vi "amoure_fast_panel.vi"() -> ()   [LabVIEW 2016]
uses:
  <vilib>/Utility/error.llb/DialogType.ctl
  states/InitializationStates.ctl
  states/DataAcqStates.ctl
  <vilib>/registry/registry.llb/Registry RtKey.ctl
  <vilib>/registry/registry.llb/Registry SAM.ctl
  <vilib>/Utility/error.llb/whitespace.ctl
  <vilib>/Analysis/baseanly.llb/Mean (DBL).vi
  <vilib>/registry/registry.llb/Read Registry Value Simple STR.vi
  Instance           5 11Saved   VFP .vi
  Instance          20 11Saved   VFP .vi
  Instance           6 11Saved   VFP .vi
  Instance          21 11Saved   VFP .vi
  Instance           8 11Saved   VFP .vi
  <vilib>/Analysis/NI_AALPro.lvlib
  <vilib>/Analysis/NI_AALBase.lvlib
panel:
  out "Target Golovochenko  (MOhm)":dbl
  in  "Applied Voltage (V)":dbl
  out "Pore Resistance":dbl
  out "Target Resistance \n(MOhm)":dbl
  out "Membrane-Solution Resistivity":dbl
  out "Membrane Resistance (MOhm)":dbl
  out "Capillary Resistance":dbl
  out "Capillary Diameter":dbl
  in  "Bare Resistance \n(MOhm)":dbl
  out "XY Graph":cluster{"type":sgl[], "type":sgl[]}(graph)
  out "Recording IV":bool
  in  "Start/Stop Saving":bool
  in  "Pick a new filename":bool
  out "Control Amp Overload":bool caption="CA"
  out "Current Overload":bool caption="I"
  out "Voltage Overload":bool caption="V"
  in  "Legacy Save":bool
  out "Front Panel Window:Title 2":string="Gamry Instruments Virtual Front Panel"
  out "Log File Refnum 2":refnum<file>
  in  "Log File 2":path
  in  "Enable Section":bool
  in  "Desired Pore Size (nm)":dbl
  in  "Membrane Thickness \n(nm)":dbl
  in  "Sealed Resistance\n(MOhm)":dbl
  in  "Solution Conductance":dbl
  in  "Smoothing Parameter":i32=100
  out "Resistance (MOhm)":dbl
  out "Current(nA)":dbl
  in  "Select Graph":u16(ring) items=["V Vs. T, I vs. T", "I vs. V", "V vs. I"]
  out "Family":string
  out "Vf History":sgl[](array[numeric])
  out "Im History":sgl[](array[numeric])
  out "XY Graph Flipped?":bool
  in  "CA Speed":u16(ring)
  in  "I/E Stability":u16(ring)=2 items=["Fast", "Medium Fast", "Normal", "Slow"]
  in  "IchOffsetEnable":bool
  in  "VchOffsetEnable":bool
  in  "Ich Offset":sgl step=0.1 format="%^.3e"
  in  "Vch Offset":sgl step=0.1 format="%^.3e"
  in  "Ich Filter":u16(ring)
  in  "Vch Filter":u16(ring)
  in  "Ich Autorange":bool
  in  "Vch Autorange":bool
  in  "I/E Autorange":bool
  in  "I/E Range":u16(ring)
  in  "Ich Range":u16(ring)
  in  "Vch Range":u16(ring)
  in  "Device":u16(ring)
  in  "CtrlMode":u32(ring)=1 items=["Galvanostat", "Potentiostat", "ZRA"]
  in  "Continuous":bool=TRUE
  in  "Acq. Frequency":dbl=100.0 caption="Hz" min=0.001667 max=300000.0 step=1.0 format="%.3f"
  in  "Cycles":u32=1 min=1 step=1
  in  "Signal Type":u16(ring) items=["Take IV Curve"=9, "Sine Wave"=0, "Cosine Wave"=1, "Triangle"=2, "Square Wave"=3, "Sawtooth"=4, "Ramp"=5, "Single Point"=7, "From File"=8]
  in  "Filename":path
  in  "Phase Offset":dbl caption="Degrees" step=1.0 format="%.3f"
  in  "DC Offset":dbl caption="V" step=0.1 format="%^.3e"
  in  "Amplitude":dbl=0.1 caption="V" step=0.1 format="%^.3e"
  in  "Signal Frequency":dbl=1.0 caption="Hz" min=5e-05 max=300000.0 step=0.5 format="%.3f"
  in  "Final":dbl=1.0 caption="V" step=0.1 format="%^.3e"
  in  "Initial":dbl caption="V" step=0.1 format="%^.3e"
  in  "Duty Cycle":dbl=50.0 caption="Percent" min=0.0 max=100.0 step=0.1 format="%.3f"
  in  "Scan Rate":dbl=1.0 caption="V/s" step=0.01 format="%_3f"
  in  "Cell State":bool
  in  "Auto Cell Switch":bool=TRUE
  in  "Start/Stop":bool caption="Start"
  out "Confirm Exit?":bool
  out "?":sgl[][](graph)
  out "I vs. V":cluster{dbl, dbl}[](graph)
  out "SetCell":bool
  out "Cell Val Change NewVal":bool
  out "Version":string
  in  "[user-defined codes]":u32[](array[numeric])=[3758096430]
  in  "[user-defined descriptions]":string[](array[string])=["Device Not Authorized"]
  out "Taking Data":bool
  out "Front Panel Window:Title":string="Gamry Instruments Virtual Front Panel"
  in  "Log File":path
  out "Device Gone":bool
  out "Index of Device (Device Change)":i32
  out "milliseconds to wait":u32=150
  in  "Close":bool
  out "From File Refnum":refnum<file>
  out "Data Handlers":T1
  out "Log File Refnum":refnum<file>
  out "ForcePstatFunctionUpdate":bool
  out "File Data":string
  out "Device List Change Callback":refnum<k27>
  in  "Device List Change":bool
  out "Device Open":bool
  out "Section":string
  in  "GAMRYCOMLib.IGamrySignalArray":refnum<k7>
  in  "GAMRYCOMLib.IGamryDtaqIv":refnum<k7>
  in  "GAMRYCOMLib.IGamryPstat":refnum<k7>
  in  "GAMRYCOMLib.IGamryDeviceList":refnum<k7>
  out "DataDone Callback":refnum<k27>
  out "DataDone?":bool
  out "Dtaq Graph Callback":refnum<k27>
  in  "GAMRYCOMLib.IGamrySignal":refnum<k7>
  out "Signal":refnum<k7>
  out "Dtaq":refnum<k7>
  out "Pstat":refnum<k7>
  out "Device List":refnum<k7>
  out "First I/E Range":i32
  out "Section List":string[](array[string])=["PC5600-00002"]
  # "amoureux"
  # "Live View"
  # "Save"
  # "Overloads"
  # "1"
  # "2"
  # "displacing carbon atoms since 2018"
  # "Signal Generation"
  # "Nanopore Creator"
  # "Device Settings"
  # "Experiment Control"
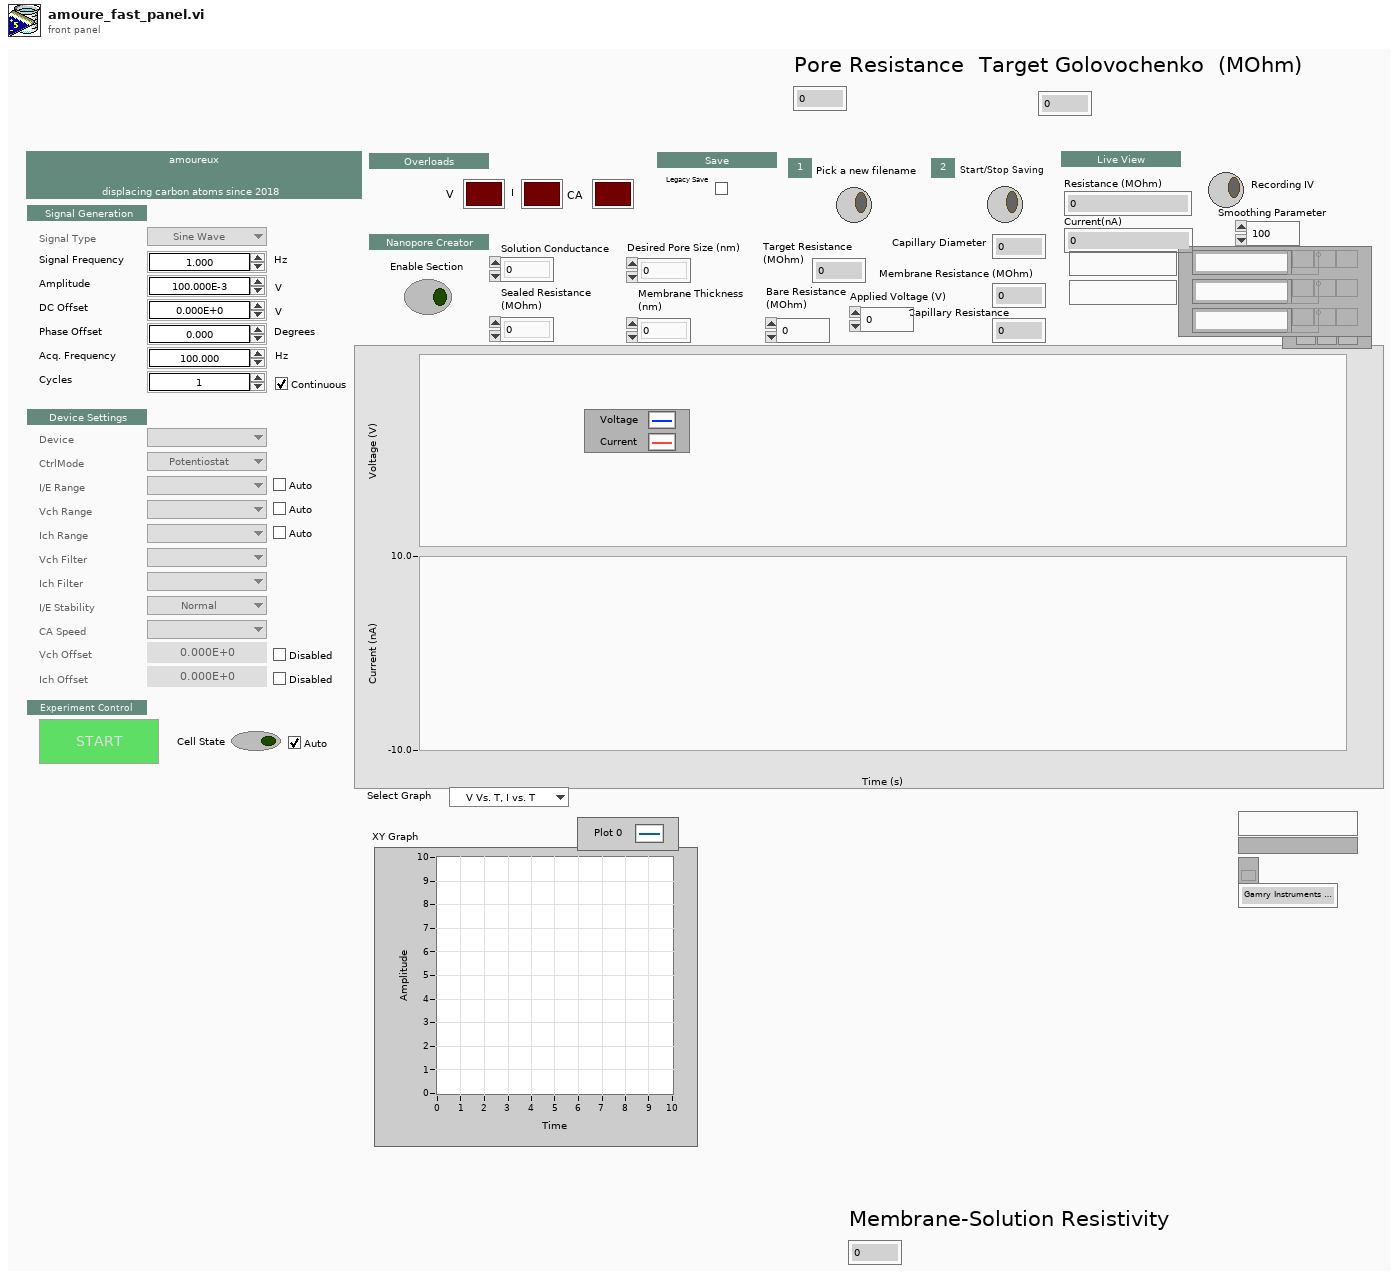
[diagram p1: front panel]
types:
  T1 = cluster{"Vs. T":refnum<vi>, "I vs. V":refnum<vi>, "Log File Refnum":refnum<vi>}
  T2 = typedef "DialogType.ctl" = u16
  T3 = enum32{"invalid app kind", "Development System", "Run Time System", "Student Edition", "Embedded LabVIEW", "Evaluation", "Custom"}
  T4 = typedef "InitializationStates.ctl" = enum16{"Initialize COM", "Load Device List", "Load Range Strings", "Setup Ranges", "Adjust Menu", "STOP"}
  T5 = typedef "DataAcqStates.ctl" = enum16{"Initialize", "Initialize Objects", "Generate Signal", "Data Acq Setup", "Acquire Data", "Cleanup", "STOP"}
  T6 = typedef "Registry SAM.ctl" = enum32{"KEY_QUERY_VALUE", "KEY_SET_VALUE", "KEY_CREATE_SUB_KEY", "KEY_ENUMERATE_SUB_KEYS", "KEY_NOTIFY", "KEY_CREATE_LINK", "KEY_READ", "KEY_WRITE", "KEY_ALL_ACCESS", "KEY_READ | KEY_WRITE"}
  T7 = typedef "Registry RtKey.ctl" = enum32{"HKEY_CLASSES_ROOT", "HKEY_CURRENT_USER", "HKEY_LOCAL_MACHINE", "HKEY_USERS", "HKEY_PERFORMANCE_DATA", "HKEY_CURRENT_CONFIG", "HKEY_DYN_DATA"}
  T8 = enum16{"open", "open or create", "create or replace", "create", "open (read only)"}
  T9 = cluster{"Ctrl Reference":refnum<vi>, "I vs. V":refnum<vi>, "Log File Refnum":refnum<vi>}
  T10 = cluster{"I/E Ranges":string[], "First I/E Range":i32, "VchRanges":string[], "IchRanges":string[], "AchRanges":string[], "VchFilters":string[], "IchFilters":string[], "AchFilters":string[], "Family":string, "CA Speeds":string[]}
  T11 = enum32{"existing file", "new file", "new or existing file", "existing dir", "new dir", "new or existing dir", "existing file (use LLBs)", "new file (use LLBs)", "new or existing file (use LLBs)", "new or existing file or directory (use LLBs)"}
  T12 = typedef "Registry refnum.ctl" = refnum<k1>
  T13 = typedef "whitespace.ctl" = u16
  T14 = cluster{"I Overload":bool, "CA Overload":bool, "V Overload":bool, "I ADC Railed":bool, "V ADC Railed":bool}
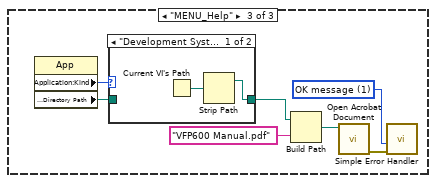
[diagram p3: hidden frame]
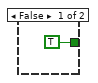
[diagram p5: hidden frame]
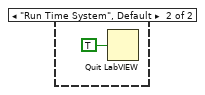
[diagram p7: hidden frame]
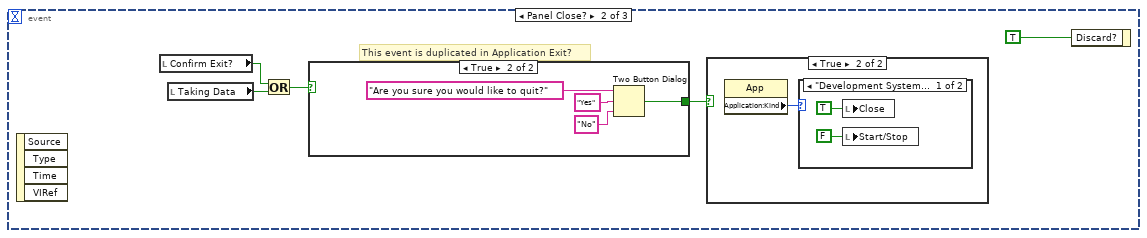
[diagram p8: hidden frame]
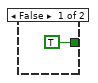
[diagram p9: hidden frame]
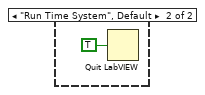
[diagram p11: hidden frame]
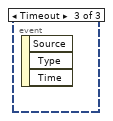
[diagram p12: hidden frame]
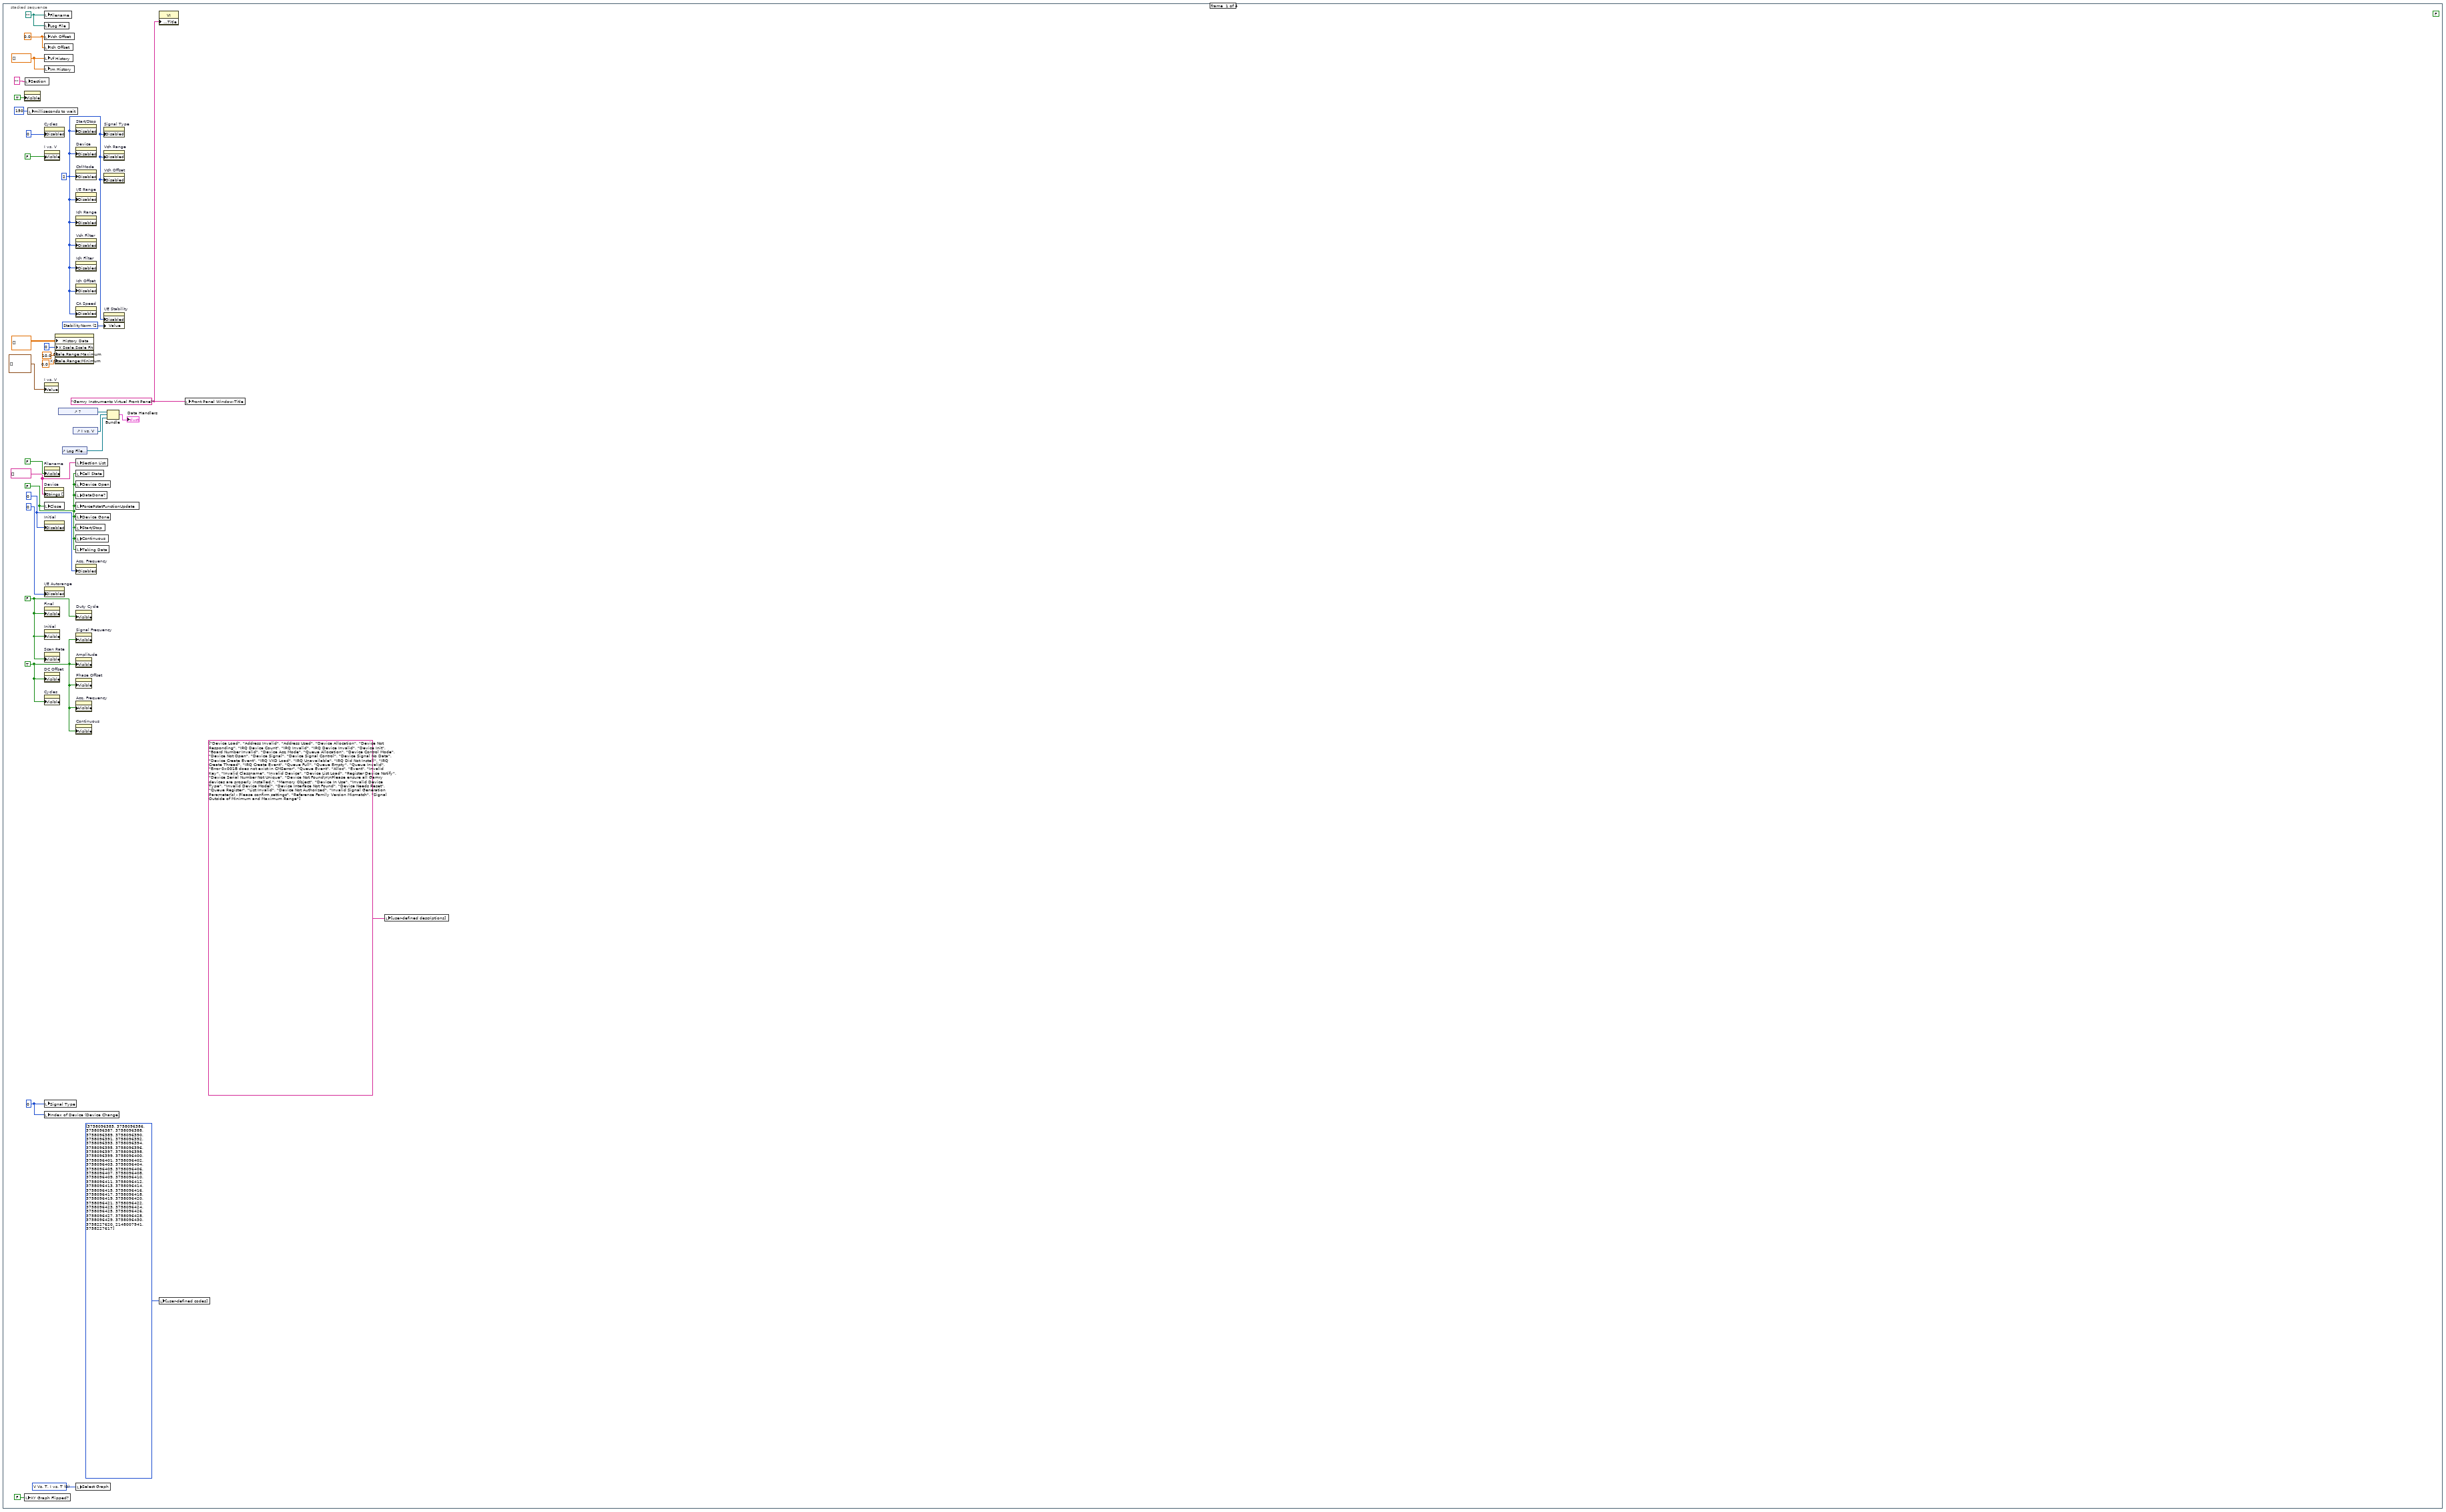
[diagram p13: hidden frame]
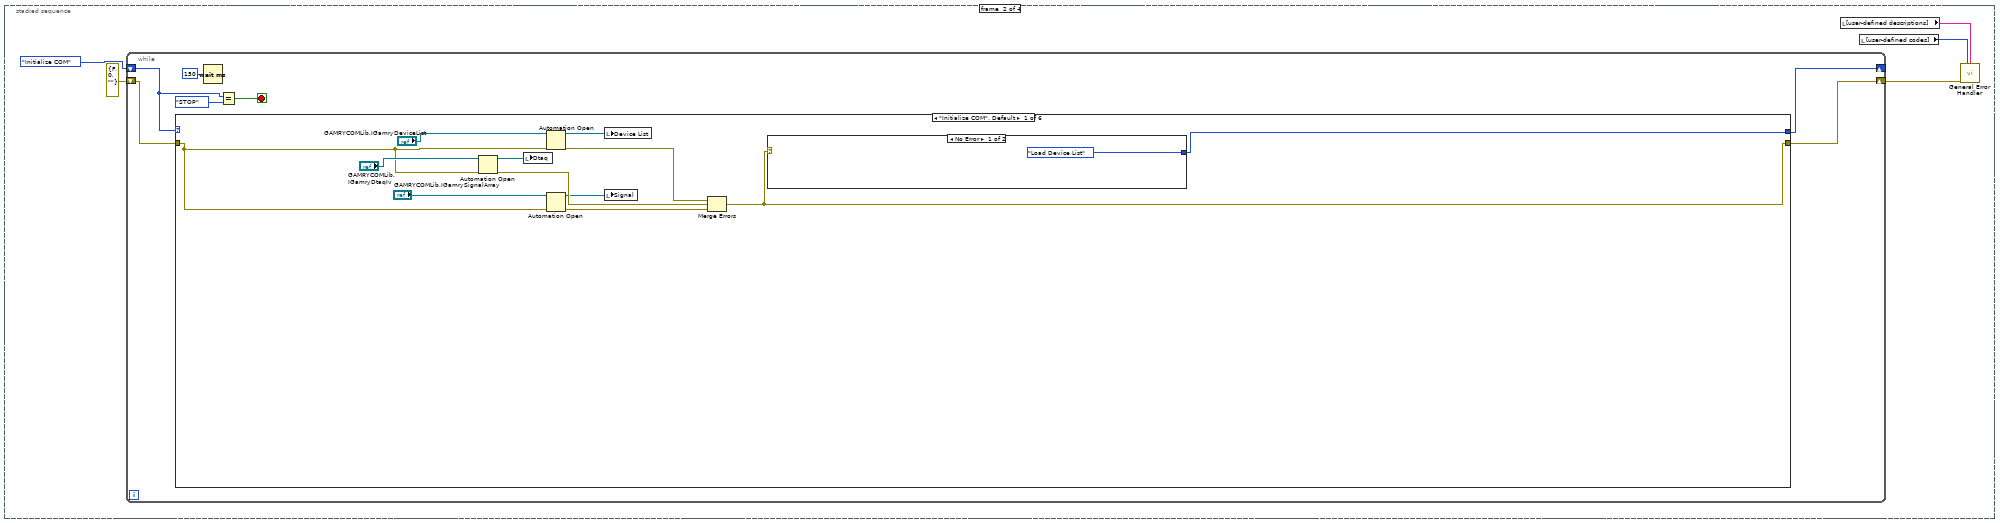
[diagram p14: hidden frame]
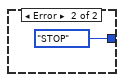
[diagram p15: hidden frame]
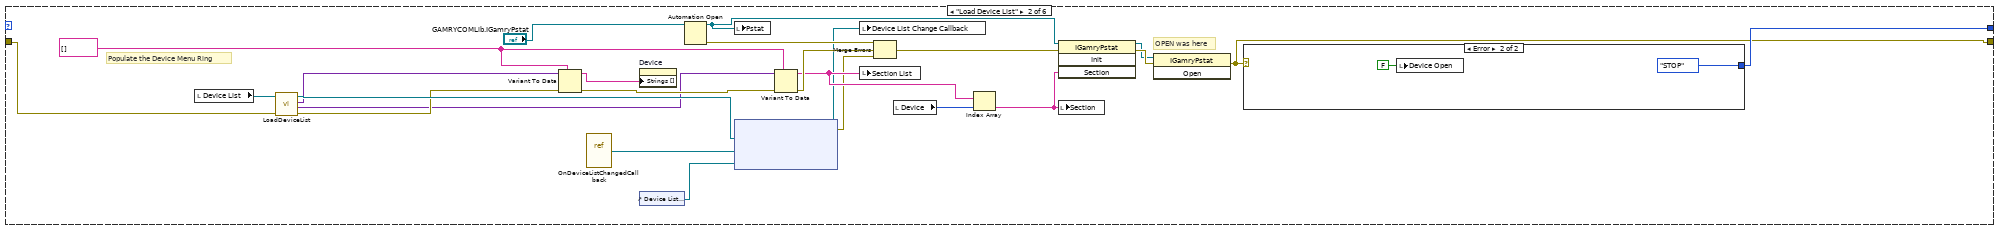
[diagram p16: hidden frame]
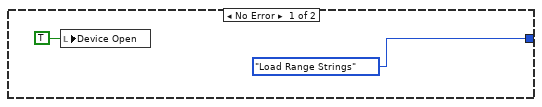
[diagram p17: hidden frame]
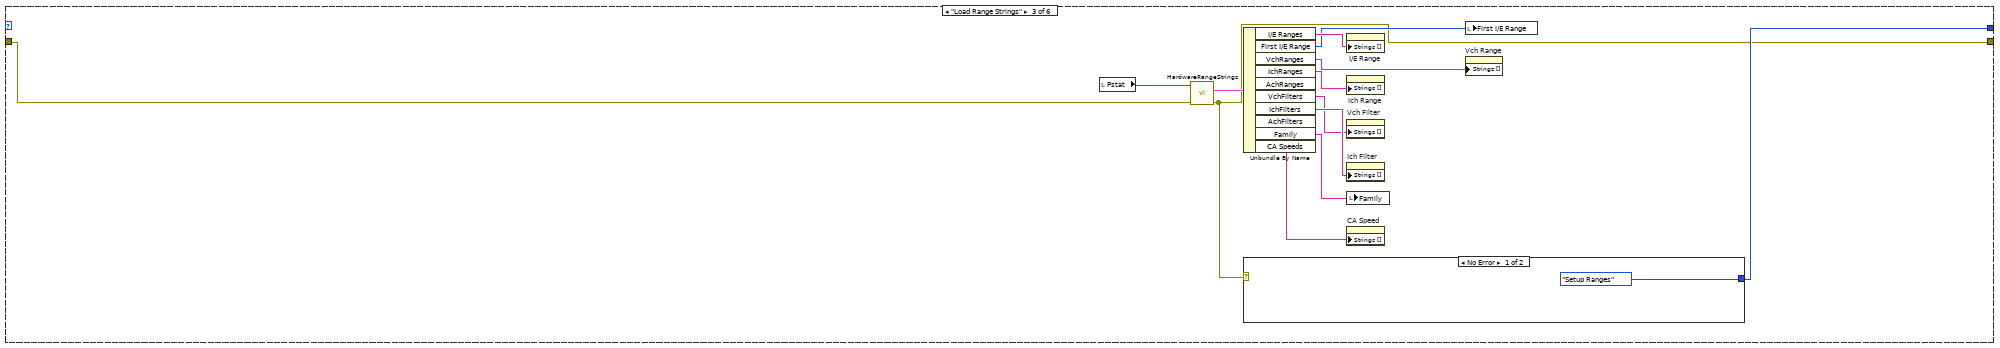
[diagram p18: hidden frame]
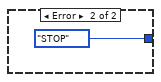
[diagram p19: hidden frame]
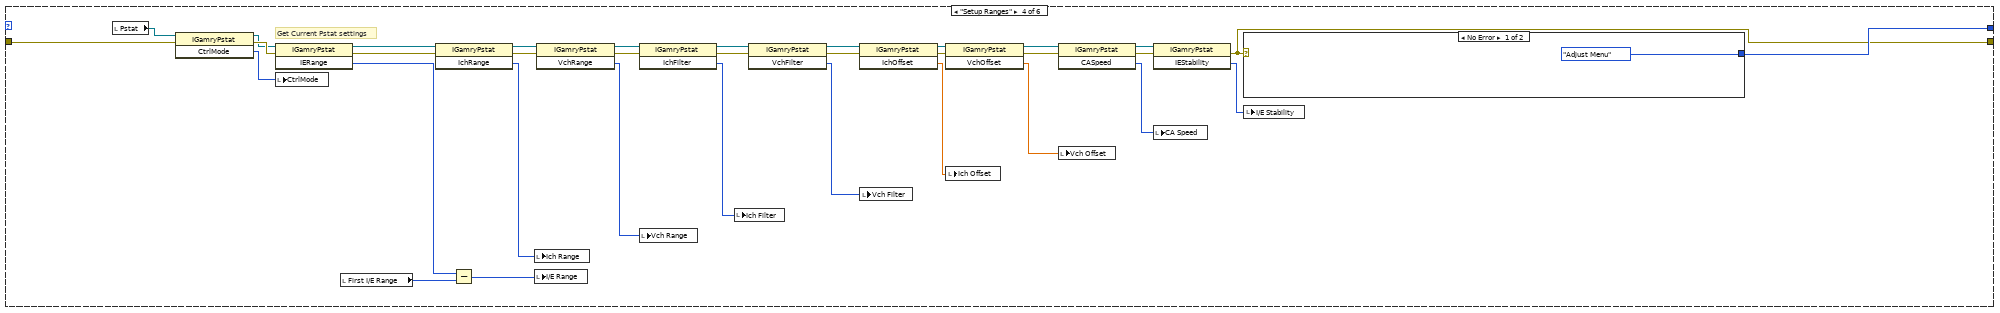
[diagram p20: hidden frame]
diagram:
  w1 = FALSE
  # "REMEMBER TO CHANGE THE VERSION NUMBER!!!!"
  # "1/600 - 4KHz"
  n1 = while {
    stop <- w7 continue-if-true
    n2 = local read "Close"() -> (w8:bool)
    n3 = local read "milliseconds to wait"() -> (w4:u32)
    n4 = Current VI's Menubar() -> (w5:refnum<k9>)
    n5 = Not(x=w8) -> (.not. x?=w7:bool)
    n6 = Get Menu Selection(0:w5) -> (6:w6:string)  [unwired: 3 in, 4 out]
    n7 = case shown="\"MENU_About_VFP\"" w6 {
      frame "False", Default {
      }
      frame "MENU_About_VFP" {
        n8 = local read "Version"() -> (w9:string)
        n9 = Concatenate Strings("Virtual Front Panel\nVersion " ("message"), w9, "\nCopyright 2010\nGamry Instruments, Inc." ("message")) -> (w12:string)
        n10 = One Button Dialog(message=w12) -> ()  [unwired: 1 in, 1 out]
      }
      frame "MENU_Help" {
        w13 = T2 1 items=["no dialog", "OK message", "continue or stop message", "OK message + warnings", "continue/stop + warnings"] ("type of dialog (OK msg:1)")
        n11 = property class="App"() -> ("Application:Kind"=w15:T3, "Application:Directory Path"=w14:path)  [unwired: 2 in, 2 out]
        n12 = case shown="\"Development System\"" w15 {
          tunnel: [w20 w22] -> w19
          tunnel: w14 -> [_ w22]
          frame "Development System" {
            n13 = Current VI's Path() -> (path=w21:path)
            n14 = Strip Path(path=w21) -> (stripped path=w20:path)  [unwired: 1 out]
          }
          frame "Run Time System", Default {
          }
        }
        n15 = Build Path(base path=w19, name or relative path="VFP600 Manual.pdf") -> (appended path=w17:path)
        n16 = call <vilib>:"Open Acrobat Document.vi"("acrobat document"=w17) -> ("error out"=w16:errorcluster)  [unwired: 6 in]
        n17 = call <vilib>:"Simple Error Handler.vi"("type of dialog (OK msg:1)"=w13, "error in (no error)"=w16) -> ()  [unwired: 3 in, 5 out]
      }
    }
    n18 = Wait (ms)(milliseconds to wait=w4) -> ()  [unwired: 1 out]
    n19 = event shown="[0] Application Instance Close?" {
      selector: _ -> [_ _ _]
      dyn-events: _ -> [_ _ _]
      timeout: w4 -> [_ _ _]
      event Application Instance Close? {
        # "This event is duplicated in Panel Close?"
        n20 = event-data() -> ()  [unwired: 1 in, 5 out]
        n21 = local read "Confirm Exit?"() -> (w25:bool)
        n22 = local read "Taking Data"() -> (w24:bool)
        n23 = Or(x=w25, y=w24) -> (x .or. y?=w23:bool)
        n24 = case shown="True" w23 {
          tunnel: [TRUE ("T button?") w29] -> w27
          frame False {
          }
          frame True {
            n25 = Two Button Dialog(message="Are you sure you would like to quit?", 1:"No" ("F button name (\"Cancel\")"), 2:"Yes" ("T button name (\"OK\")")) -> (T button?=w29:bool)
          }
        }
        n26 = case shown="True" w27 {
          frame False {
          }
          frame True {
            n27 = property class="App"() -> ("Application:Kind"=w33:T3)  [unwired: 2 in, 2 out]
            n28 = case shown="\"Development System\"" w33 {
              frame "Development System" {
                n29 = local write "Close"(TRUE) -> ()
                n30 = local write "Start/Stop"(FALSE) -> ()
              }
              frame "Run Time System", Default {
                n31 = Quit LabVIEW(quit? (T)=TRUE) -> ()
              }
            }
          }
        }
        n32 = event-data("Discard?"=TRUE) -> ()  [unwired: 2 in, 1 out]
      }
      event Panel Close? {
        # "This event is duplicated in Application Exit?"
        n33 = event-data() -> ()  [unwired: 1 in, 4 out]
        n34 = local read "Confirm Exit?"() -> (w39:bool)
        n35 = local read "Taking Data"() -> (w38:bool)
        n36 = Or(x=w39, y=w38) -> (x .or. y?=w37:bool)
        n37 = case shown="True" w37 {
          tunnel: [TRUE ("T button?") w43] -> w41
          frame False {
          }
          frame True {
            n38 = Two Button Dialog(message="Are you sure you would like to quit?", 1:"No" ("F button name (\"Cancel\")"), 2:"Yes" ("T button name (\"OK\")")) -> (T button?=w43:bool)
          }
        }
        n39 = case shown="True" w41 {
          frame False {
          }
          frame True {
            n40 = property class="App"() -> ("Application:Kind"=w47:T3)  [unwired: 2 in, 2 out]
            n41 = case shown="\"Development System\"" w47 {
              frame "Development System" {
                n42 = local write "Close"(TRUE) -> ()
                n43 = local write "Start/Stop"(FALSE) -> ()
              }
              frame "Run Time System", Default {
                n44 = Quit LabVIEW(quit? (T)=TRUE) -> ()
              }
            }
          }
        }
        n45 = event-data("Discard?"=TRUE) -> ()  [unwired: 1 in, 1 out]
      }
      event Timeout {
        n46 = event-data() -> ()  [unwired: 1 in, 3 out]
      }
    }
  }
  n47 = stacked-sequence {
    frame #0 {
      w52 = sgl[] [] ("Vf History")
      w54 = u16 0 items=["V Vs. T, I vs. T", "I vs. V", "V vs. I"] ("Select Graph")
      w59 = path ""
      w60 = 2 items=["StabilityFast", "StabilityMedFast", "StabilityNorm", "StabilitySlow"] ("Stability")
      w67 = "Gamry Instruments Virtual Front Panel" ("Front Panel Window:Title")
      w62 = FALSE ("Visible")
      w55 = u8 0 ("Disabled")
      w61 = u8 2 ("Disabled")
      (unwired) FALSE ("Visible")
      w77 = TRUE ("Visible")
      w81 = sgl 0.0 ("Vch Offset")
      w66 = FALSE ("I/E Autorange 2")
      w71 = u32 0 ("Zero")
      w72 = string[] [] ("Strings []")
      n48 = property class="WFChart (strict)"("Visible"=TRUE) -> ()  [unwired: 2 in, 2 out]
      n49 = local write "XY Graph Flipped?"(FALSE ("XY Graph Flipped?")) -> ()
      n50 = local write "Section"("" ("Section")) -> ()
      n51 = local write "milliseconds to wait"(u32 150 ("milliseconds to wait")) -> ()
      n52 = local write "Filename"(w59) -> ()
      n53 = local write "Log File"(w59) -> ()
      n54 = local write "Vch Offset"(w81) -> ()
      n55 = local write "Ich Offset"(w81) -> ()
      n56 = local write "Vf History"(w52) -> ()
      n57 = local write "Im History"(w52) -> ()
      n58 = property on="Cycles" class="DigNum (strict)"("Disabled"=0) -> ()  [unwired: 2 in, 2 out]
      n59 = property on="I vs. V" class="XYGraph (strict)"("Visible"=FALSE) -> ()  [unwired: 2 in, 2 out]
      n60 = property on="I vs. V" class="XYGraph (strict)"("Value"=cluster{dbl, dbl}[] [] ("I vs. V")) -> ()  [unwired: 2 in, 2 out]
      n61 = property on="Filename" class="Path"("Visible"=FALSE) -> ()  [unwired: 2 in, 2 out]
      n62 = property on="Device" class="Ring (strict)"("Strings []"=w72) -> ()  [unwired: 2 in, 2 out]
      n63 = local write "Close"(w66) -> ()
      n64 = property on="Initial" class="DigNum (strict)"("Disabled"=w55) -> ()  [unwired: 2 in, 2 out]
      n65 = property on="I/E Autorange" class="Bool (strict)"("Disabled"=u8 0) -> ()  [unwired: 2 in, 2 out]
      n66 = property on="Final" class="DigNum (strict)"("Visible"=w62) -> ()  [unwired: 2 in, 2 out]
      n67 = property on="Initial" class="DigNum (strict)"("Visible"=w62) -> ()  [unwired: 2 in, 2 out]
      n68 = property on="Scan Rate" class="DigNum (strict)"("Visible"=w62) -> ()  [unwired: 2 in, 2 out]
      n69 = property on="DC Offset" class="DigNum (strict)"("Visible"=w77) -> ()  [unwired: 2 in, 2 out]
      n70 = property on="Cycles" class="DigNum (strict)"("Visible"=w77) -> ()  [unwired: 2 in, 2 out]
      n71 = local write "Signal Type"(w71) -> ()
      n72 = local write "Index of Device (Device Change)"(w71) -> ()
      n73 = property class="WFChart (strict)"("History Data"=sgl[][] [], "X Scale.Scale Fit"=u8 0, "X Scale.Range:Maximum"=10.0, "X Scale.Range:Minimum"=0.0) -> ()  [unwired: 2 in, 2 out]
      n74 = control-ref of="?"() -> (w80:refnum<vi>)
      n75 = control-ref of="Log File Refnum"() -> (w75:refnum<vi>)
      n76 = control-ref of="I vs. V"() -> (w79:refnum<vi>)
      n77 = property on="Start/Stop" class="Bool (strict)"("Disabled"=w61) -> ()  [unwired: 2 in, 2 out]
      n78 = property on="Device" class="Ring (strict)"("Disabled"=w61) -> ()  [unwired: 2 in, 2 out]
      n79 = property on="CtrlMode" class="Ring (strict)"("Disabled"=w61) -> ()  [unwired: 2 in, 2 out]
      n80 = property on="I/E Range" class="Ring (strict)"("Disabled"=w61) -> ()  [unwired: 2 in, 2 out]
      n81 = property on="Ich Range" class="Ring (strict)"("Disabled"=w61) -> ()  [unwired: 2 in, 2 out]
      n82 = property on="Vch Filter" class="Ring (strict)"("Disabled"=w61) -> ()  [unwired: 2 in, 2 out]
      n83 = property on="Ich Filter" class="Ring (strict)"("Disabled"=w61) -> ()  [unwired: 2 in, 2 out]
      n84 = property on="Ich Offset" class="DigNum (strict)"("Disabled"=w61) -> ()  [unwired: 2 in, 2 out]
      n85 = property on="CA Speed" class="Ring (strict)"("Disabled"=w61) -> ()  [unwired: 2 in, 2 out]
      n86 = local write "Section List"(w72) -> ()
      n87 = local write "Cell State"(w66) -> ()
      n88 = local write "Device Open"(w66) -> ()
      n89 = local write "DataDone?"(w66) -> ()
      n90 = local write "ForcePstatFunctionUpdate"(w66) -> ()
      n91 = local write "Device Gone"(w66) -> ()
      n92 = local write "Start/Stop"(w66) -> ()
      n93 = local write "Continuous"(w66) -> ()
      n94 = local write "Taking Data"(w66) -> ()
      n95 = property on="Acq. Frequency" class="DigNum (strict)"("Disabled"=w55) -> ()  [unwired: 2 in, 2 out]
      n96 = property on="Duty Cycle" class="DigNum (strict)"("Visible"=w62) -> ()  [unwired: 2 in, 2 out]
      n97 = property on="Signal Frequency" class="DigNum (strict)"("Visible"=w77) -> ()  [unwired: 2 in, 2 out]
      n98 = property on="Amplitude" class="DigNum (strict)"("Visible"=w77) -> ()  [unwired: 2 in, 2 out]
      n99 = property on="Phase Offset" class="DigNum (strict)"("Visible"=w77) -> ()  [unwired: 2 in, 2 out]
      n100 = property on="Acq. Frequency" class="DigNum (strict)"("Visible"=w77) -> ()  [unwired: 2 in, 2 out]
      n101 = property on="Continuous" class="Bool (strict)"("Visible"=w77) -> ()  [unwired: 2 in, 2 out]
      n102 = local write "Select Graph"(w54) -> ()
      n103 = property on="Signal Type" class="Ring (strict)"("Disabled"=w61) -> ()  [unwired: 2 in, 2 out]
      n104 = property on="Vch Range" class="Ring (strict)"("Disabled"=w61) -> ()  [unwired: 2 in, 2 out]
      n105 = property on="Vch Offset" class="DigNum (strict)"("Disabled"=w61) -> ()  [unwired: 2 in, 2 out]
      n106 = property on="I/E Stability" class="Ring (strict)"("Disabled"=w61, "Value"=w60) -> ()  [unwired: 2 in, 2 out]
      n107 = Bundle("Ctrl Reference"=w80, "I vs. V"=w79, "Log File Refnum"=w75) -> (→"Data Handlers":T9)  [unwired: 1 in]
      n108 = property class="VI"("Front Panel Window:Title"=w67) -> ()  [unwired: 2 in, 2 out]
      n109 = local write "[user-defined codes]"(u32[] [3758096385, 3758096386, 3758096387, 3758096388, 3758096389, 3758096390, 3758096391, 3758096392, 3758096393, 3758096394, 3758096395, 3758096396, 3758096397, 3758096398, 3758096399, 3758096400, 3758096401, 3758096402, 3758096403, 3758096404, 3758096405, 3758096406, 3758096407, 3758096408, 3758096409, 3758096410, 3758096411, 3758096412, 3758096413, 3758096414, 3758096415, 3758096416, 3758096417, 3758096418, 3758096419, 3758096420, 3758096421, 3758096422, 3758096423, 3758096424, 3758096425, 3758096426, 3758096427, 3758096428, 3758096429, 3758096430, 3758227620, 2148007941, 3758227617] ("[user-defined codes]")) -> ()
      n110 = local write "Front Panel Window:Title"(w67) -> ()
      n111 = local write "[user-defined descriptions]"(string[] ["Device Load", "Address Invalid", "Address Used", "Device Allocation", "Device Not Responding", "IRQ Device Count", "IRQ Invalid", "IRQ Device Invalid", "Device Init", "Board Number Invalid", "Device Acq Mode", "Queue Allocation", "Device Control Mode", "Device Not Open", "Device Signal", "Device Signal Control", "Device Signal No Data", "Device Create Event", "IRQ VXD Load", "IRQ Unavailable", "IRQ Did Not Install", "IRQ Create Thread", "IRQ Create Event", "Queue Full", "Queue Empty", "Queue Invalid", "Error 0x001B does not exist in CMSerror", "Queue Event", "Alloc", "Event", "Invalid Key", "Invalid Classname", "Invalid Device", "Device List Load", "Register Device Notify", "Device Serial Number Not Unique", "Device Not Found\n\nPlease ensure all Gamry devices are properly installed.", "Memory Object", "Device In Use", "Invalid Device Type", "Invalid Device Model", "Device Interface Not Found", "Device Needs Reset", "Queue Register", "List Invalid", "Device Not Authorized", "Invalid Signal Generation Parameter(s) - Please confirm settings", "Reference Family Version Mismatch", "Signal Outside of Minimum and Maximum Range"] ("[user-defined descriptions]")) -> ()
    }
    frame #1 {
      n112 = while {
        shift-right: [w88] -> _
        shift-left: InitializationStates."Initialize COM" ("Initialization States") -> [w94]
        shift-right: [w90] -> w83
        shift-left: errorcluster {"status"=FALSE, "code"=0, "source"=""} ("error out") -> [w89]
        stop <- w92 stop-if-true
        n113 = case shown="\"Initialize COM\", Default" w94 {
          tunnel: [w96 w109 w138 w153 w189 w208] -> w90
          tunnel: w89 -> [w97 w114 w140 w180 w190 w208]
          tunnel: [w95 w112 w144 w179 w198 InitializationStates."STOP" ("Initialization States")] -> w88
          frame "Initialize COM", Default {
            n114 = Automation Open(error in (no error)=w97, Automation Refnum="GAMRYCOMLib.IGamryDtaqIv") -> (Automation Refnum=w98:refnum<k7>, error out=w104:errorcluster)  [unwired: 2 in]
            n115 = local write "Dtaq"(w98) -> ()
            n116 = Automation Open(error in (no error)=w97, Automation Refnum="GAMRYCOMLib.IGamryDeviceList") -> (Automation Refnum=w106:refnum<k7>, error out=w103:errorcluster)  [unwired: 2 in]
            n117 = Automation Open(error in (no error)=w97, Automation Refnum="GAMRYCOMLib.IGamrySignalArray") -> (Automation Refnum=w99:refnum<k7>, error out=w105:errorcluster)  [unwired: 2 in]
            n118 = local write "Device List"(w106) -> ()
            n119 = local write "Signal"(w99) -> ()
            n120 = Merge Errors(w103, w104, w105) -> (w96:errorcluster)
            n121 = case shown="No Error" w96 {
              tunnel: [InitializationStates."Load Device List" ("Initialization States") InitializationStates."STOP" ("Initialization States")] -> w95
              frame No Error {
              }
              frame Error {
              }
            }
          }
          frame "Load Device List" {
            w116 = string[] []
            # "OPEN was here"
            # "Populate the Device Menu Ring"
            n122 = local read "Device List"() -> (w133:refnum<k7>)
            n123 = call "LoadDeviceList.vi"("Error In"=w114, "GAMRYCOMLib.IGamryDeviceList In"=w133) -> ("Error Out"=w129:errorcluster, "EnumSections"=w128:variant, "EnumLabels"=w127:variant, "GAMRYCOMLib.IGamryDeviceList Out"=w132:refnum<k7>)  [unwired: 4 in]
            n124 = Variant To Data(error in=w129, type=w116, Variant=w127) -> (data=w115:string[], error out=w131:errorcluster)
            n125 = vi-ref "OnDeviceListChangedCallback.vi"() -> ("vi reference"=w122:refnum<vi>)
            n126 = property on="Device" class="Ring (strict)"("Strings []"=w115) -> ()  [unwired: 2 in, 2 out]
            n127 = control-ref of="Device List Change"() -> (w121:refnum<vi>)
            n128 = Automation Open(Automation Refnum="GAMRYCOMLib.IGamryPstat") -> (Automation Refnum=w120:refnum<k7>, error out=w125:errorcluster)  [unwired: 3 in]
            n129 = local write "Pstat"(w120) -> ()
            n130 = node(w132, w122, w121) -> (w123:refnum<k27>, w113:errorcluster)  [unwired: 2 in]
            n131 = Variant To Data(error in=w131, type=w116, Variant=w128) -> (data=w124:string[], error out=w130:errorcluster)
            n132 = local write "Device List Change Callback"(w123) -> ()
            n133 = local write "Section List"(w124) -> ()
            n134 = Merge Errors(w125, w130, w113) -> (w126:errorcluster)
            n135 = local read "Device"() -> (w118:u16)
            n136 = Index Array(array=w124, index=w118) -> (element=w119:string)
            n137 = invoke class="IGamryPstat" method="Init"(reference=w120, error in=w126, "Section"=w119) -> (reference out=w110:refnum<k7>, error out=w111:errorcluster)  [unwired: 1 in, 2 out]
            n138 = local write "Section"(w119) -> ()
            n139 = invoke class="IGamryPstat" method="Open"(reference=w110, error in=w111) -> (error out=w109:errorcluster)  [unwired: 1 in, 2 out]
            n140 = case shown="Error" w109 {
              tunnel: [InitializationStates."Load Range Strings" ("Initialization States") InitializationStates."STOP" ("Initialization States")] -> w112
              frame No Error {
                n141 = local write "Device Open"(TRUE ("Device Open")) -> ()
              }
              frame Error {
                n142 = local write "Device Open"(FALSE ("Device Open")) -> ()
              }
            }
          }
          frame "Load Range Strings" {
            n143 = local read "Pstat"() -> (w141:refnum<k7>)
            n144 = call "HardwareRangeStrings.vi"("error in (no error)"=w140, "Pstat IN"=w141) -> ("error out"=w138:errorcluster, "Hardware Strings"=w139:T10)  [unwired: 7 in, 1 out]
            n145 = Unbundle By Name(w139) -> ("I/E Ranges"=w148:string[], "First I/E Range"=w145:i32, "VchRanges"=w146:string[], "IchRanges"=w147:string[], "VchFilters"=w149:string[], "IchFilters"=w150:string[], "Family"=w142:string, "CA Speeds"=w143:string[])  [unwired: 2 out]
            n146 = case shown="No Error" w138 {
              tunnel: [InitializationStates."Setup Ranges" ("Initialization States") InitializationStates."STOP" ("Initialization States")] -> w144
              frame No Error {
              }
              frame Error {
              }
            }
            n147 = property on="I/E Range" class="Ring (strict)"("Strings []"=w148) -> ()  [unwired: 2 in, 2 out]
            n148 = property on="Ich Range" class="Ring (strict)"("Strings []"=w147) -> ()  [unwired: 2 in, 2 out]
            n149 = property on="Vch Filter" class="Ring (strict)"("Strings []"=w149) -> ()  [unwired: 2 in, 2 out]
            n150 = property on="Ich Filter" class="Ring (strict)"("Strings []"=w150) -> ()  [unwired: 2 in, 2 out]
            n151 = local write "Family"(w142) -> ()
            n152 = property on="CA Speed" class="Ring (strict)"("Strings []"=w143) -> ()  [unwired: 2 in, 2 out]
            n153 = local write "First I/E Range"(w145) -> ()
            n154 = property on="Vch Range" class="Ring (strict)"("Strings []"=w146) -> ()  [unwired: 2 in, 2 out]
          }
          frame "Setup Ranges" {
            # "Get Current Pstat settings"
            n155 = local read "Pstat"() -> (w181:refnum<k7>)
            n156 = invoke class="IGamryPstat" method="CtrlMode"(reference=w181, error in=w180) -> (reference out=w185:refnum<k7>, error out=w186:errorcluster, "CtrlMode"=w183:i32)  [unwired: 1 in]
            n157 = invoke class="IGamryPstat" method="IERange"(reference=w185, error in=w186) -> (reference out=w155:refnum<k7>, error out=w154:errorcluster, "IERange"=w182:i32)  [unwired: 1 in]
            n158 = local write "CtrlMode"(w183) -> ()
            n159 = local read "First I/E Range"() -> (w178:i32)
            n160 = invoke class="IGamryPstat" method="IchRange"(reference=w155, error in=w154) -> (reference out=w160:refnum<k7>, error out=w159:errorcluster, "IchRange"=w157:i32)  [unwired: 1 in]
            n161 = Subtract(x=w182, y=w178) -> (x-y=w184:i32)
            n162 = local write "Ich Range"(w157) -> ()
            n163 = local write "I/E Range"(w184) -> ()
            n164 = invoke class="IGamryPstat" method="VchRange"(reference=w160, error in=w159) -> (reference out=w173:refnum<k7>, error out=w156:errorcluster, "VchRange"=w158:i32)  [unwired: 1 in]
            n165 = invoke class="IGamryPstat" method="IchFilter"(reference=w173, error in=w156) -> (reference out=w168:refnum<k7>, error out=w167:errorcluster, "IchFilter"=w169:i32)  [unwired: 1 in]
            n166 = local write "Vch Range"(w158) -> ()
            n167 = local write "Ich Filter"(w169) -> ()
            n168 = invoke class="IGamryPstat" method="VchFilter"(reference=w168, error in=w167) -> (reference out=w175:refnum<k7>, error out=w174:errorcluster, "VchFilter"=w170:i32)  [unwired: 1 in]
            n169 = invoke class="IGamryPstat" method="IchOffset"(reference=w175, error in=w174) -> (reference out=w165:refnum<k7>, error out=w166:errorcluster, "IchOffset"=w171:sgl)  [unwired: 1 in]
            n170 = local write "Vch Filter"(w170) -> ()
            n171 = invoke class="IGamryPstat" method="VchOffset"(reference=w165, error in=w166) -> (reference out=w177:refnum<k7>, error out=w176:errorcluster, "VchOffset"=w172:sgl)  [unwired: 1 in]
            n172 = local write "Ich Offset"(w171) -> ()
            n173 = invoke class="IGamryPstat" method="CASpeed"(reference=w177, error in=w176) -> (reference out=w161:refnum<k7>, error out=w162:errorcluster, "CASpeed"=w164:i32)  [unwired: 1 in]
            n174 = local write "Vch Offset"(w172) -> ()
            n175 = invoke class="IGamryPstat" method="IEStability"(reference=w161, error in=w162) -> (error out=w153:errorcluster, "IEStability"=w163:i32)  [unwired: 1 in, 1 out]
            n176 = local write "CA Speed"(w164) -> ()
            n177 = case shown="No Error" w153 {
              tunnel: [InitializationStates."Adjust Menu" ("Initialization States") InitializationStates."STOP" ("Initialization States")] -> w179
              frame No Error {
              }
              frame Error {
              }
            }
            n178 = local write "I/E Stability"(w163) -> ()
          }
          frame "Adjust Menu" {
            n179 = local read "CtrlMode"() -> (w197:u32)
            n180 = case shown="1, Default" w197 {
              tunnel: ["V" ("Caption.Text") "A" ("Caption.Text")] -> w196
              tunnel: ["V/s" ("Caption.Text") "A/s" ("Caption.Text")] -> w195
              frame 1, Default {
              }
              frame 0 {
              }
            }
            n181 = property on="Amplitude" class="DigNum (strict)"(error in=w190, "Caption.Text"=w196) -> (error out=w194:errorcluster)  [unwired: 1 in, 1 out]
            n182 = property on="DC Offset" class="DigNum (strict)"(error in=w194, "Caption.Text"=w196) -> (error out=w193:errorcluster)  [unwired: 1 in, 1 out]
            n183 = property on="Initial" class="DigNum (strict)"(error in=w193, "Caption.Text"=w196) -> (error out=w192:errorcluster)  [unwired: 1 in, 1 out]
            n184 = property on="Final" class="DigNum (strict)"(error in=w192, "Caption.Text"=w196) -> (error out=w191:errorcluster)  [unwired: 1 in, 1 out]
            n185 = property on="Scan Rate" class="DigNum (strict)"(error in=w191, "Caption.Text"=w195) -> (error out=w189:errorcluster)  [unwired: 1 in, 1 out]
            n186 = case shown="No Error" w189 {
              tunnel: [InitializationStates."STOP" ("Initialization States") InitializationStates."STOP" ("Initialization States")] -> w198
              frame No Error {
                w203 = u8 0 ("Disabled")
                # "Enable appropriate menu stuff"
                n187 = property on="Ich Offset" class="DigNum (strict)"("Disabled"=w203) -> ()  [unwired: 2 in, 2 out]
                n188 = property on="Device" class="Ring (strict)"("Disabled"=w203) -> ()  [unwired: 2 in, 2 out]
                n189 = property on="Ich Range" class="Ring (strict)"("Disabled"=w203) -> ()  [unwired: 2 in, 2 out]
                n190 = property on="CtrlMode" class="Ring (strict)"("Disabled"=w203) -> ()  [unwired: 2 in, 2 out]
                n191 = property on="CA Speed" class="Ring (strict)"("Disabled"=w203) -> ()  [unwired: 2 in, 2 out]
                n192 = property on="Ich Filter" class="Ring (strict)"("Disabled"=w203) -> ()  [unwired: 2 in, 2 out]
                n193 = property on="Start/Stop" class="Bool (strict)"("Disabled"=w203) -> ()  [unwired: 2 in, 2 out]
                n194 = property on="I/E Range" class="Ring (strict)"("Disabled"=w203) -> ()  [unwired: 2 in, 2 out]
                n195 = property on="I/E Stability" class="Ring (strict)"("Disabled"=w203) -> ()  [unwired: 2 in, 2 out]
                n196 = property on="Vch Offset" class="DigNum (strict)"("Disabled"=w203) -> ()  [unwired: 2 in, 2 out]
                n197 = property on="Vch Range" class="Ring (strict)"("Disabled"=w203) -> ()  [unwired: 2 in, 2 out]
                n198 = property on="Signal Type" class="Ring (strict)"("Disabled"=w203) -> ()  [unwired: 2 in, 2 out]
                n199 = property on="Vch Filter" class="Ring (strict)"("Disabled"=w203) -> ()  [unwired: 2 in, 2 out]
              }
              frame Error {
                w207 = u16 0 items=[""] ("Device")
                w205 = u8 2 ("Disabled")
                # "Disable appropriate menu stuff"
                n200 = property on="Ich Offset" class="DigNum (strict)"("Disabled"=w205) -> ()  [unwired: 2 in, 2 out]
                n201 = property on="CtrlMode" class="Ring (strict)"("Disabled"=w205) -> ()  [unwired: 2 in, 2 out]
                n202 = property on="CA Speed" class="Ring (strict)"("Disabled"=w205) -> ()  [unwired: 2 in, 2 out]
                n203 = property on="Start/Stop" class="Bool (strict)"("Disabled"=w205) -> ()  [unwired: 2 in, 2 out]
                n204 = property on="I/E Range" class="Ring (strict)"("Disabled"=w205, "Value"=w207) -> ()  [unwired: 2 in, 2 out]
                n205 = property on="Ich Filter" class="Ring (strict)"("Disabled"=w205, "Value"=w207) -> ()  [unwired: 2 in, 2 out]
                n206 = property on="Device" class="Ring (strict)"("Disabled"=w205, "Value"=w207) -> ()  [unwired: 2 in, 2 out]
                n207 = property on="Ich Range" class="Ring (strict)"("Disabled"=w205, "Value"=w207) -> ()  [unwired: 2 in, 2 out]
                n208 = property on="I/E Stability" class="Ring (strict)"("Disabled"=w205) -> ()  [unwired: 2 in, 2 out]
                n209 = property on="Vch Range" class="Ring (strict)"("Disabled"=w205, "Value"=w207) -> ()  [unwired: 2 in, 2 out]
                n210 = property on="Vch Offset" class="DigNum (strict)"("Disabled"=w205) -> ()  [unwired: 2 in, 2 out]
                n211 = property on="Vch Filter" class="Ring (strict)"("Disabled"=w205, "Value"=w207) -> ()  [unwired: 2 in, 2 out]
              }
            }
          }
          frame "STOP" {
          }
        }
        n212 = Wait (ms)(milliseconds to wait=u32 150) -> ()  [unwired: 1 out]
        n213 = Equal?(x=w94, y=InitializationStates."STOP" ("Initialization States")) -> (x = y?=w92:bool)
      }
      n214 = local read "[user-defined descriptions]"() -> (w87:string[])
      n215 = local read "[user-defined codes]"() -> (w86:u32[])
      n216 = call <vilib>:"General Error Handler.vi"("[user-defined codes]"=w86, "[user-defined descriptions]"=w87, "error in (no error)"=w83) -> ()  [unwired: 8 in, 5 out]
    }
    frame #2 {
      n217 = while {
        stop <- w211 continue-if-true
        n218 = local read "Close"() -> (w212:bool)
        n219 = local read "milliseconds to wait"() -> (w210:u32)
        n220 = Not(x=w212) -> (.not. x?=w211:bool)
        n221 = event shown="[4] \"Cycles\", \"Signal Type\", \"Acq. Frequency\", \"Signal Frequency\", \"Amplitude\", \"DC Offset\", \"Phase Offset\", \"Initial\", \"Final\", \"Scan Rate\", \"Continuous\", \"Duty Cycle\": Value Change" {
          selector: _ -> [_ _ _ _ _ _ _ _]
          dyn-events: _ -> [_ _ _ _ _ _ _ _]
          timeout: w210 -> [_ _ _ _ _ _ _ _]
          event Timeout {
            w214 = u32 2 items=["Galvanostat", "Potentiostat", "ZRA"] ("CtrlMode")
            n222 = event-data() -> ()  [unwired: 1 in, 2 out]
            n223 = local read "Taking Data"() -> (w223:bool)
            n224 = local read "CtrlMode"() -> (w213:u32)
            n225 = local read "Family"() -> (w215:string)
            n226 = case shown="True" w223 {
              frame False {
              }
              frame True {
                n227 = local read "Vch Autorange"() -> (w226:bool)
                n228 = local read "Ich Autorange"() -> (w227:bool)
                n229 = local read "I/E Autorange"() -> (w225:bool)
                n230 = local read "Pstat"() -> (w224:refnum<k7>)
                n231 = case shown="False" w227 {
                  tunnel: w224 -> [_ w248]
                  frame False {
                    n232 = property on="Ich Range" class="Ring (strict)"("Disabled"=0) -> ()  [unwired: 2 in, 2 out]
                  }
                  frame True {
                    n233 = invoke class="IGamryPstat" method="IchRange"(reference=w248) -> ("IchRange"=w247:i32)  [unwired: 2 in, 2 out]
                    n234 = property on="Ich Range" class="Ring (strict)"("Value"=w247, "Disabled"=1) -> ()  [unwired: 2 in, 2 out]
                  }
                }
                n235 = case shown="False" w226 {
                  tunnel: w224 -> [_ w244]
                  frame False {
                    n236 = property on="Vch Range" class="Ring (strict)"("Disabled"=0) -> ()  [unwired: 2 in, 2 out]
                  }
                  frame True {
                    n237 = invoke class="IGamryPstat" method="VchRange"(reference=w244) -> ("VchRange"=w243:i32)  [unwired: 2 in, 2 out]
                    n238 = property on="Vch Range" class="Ring (strict)"("Value"=w243, "Disabled"=1) -> ()  [unwired: 2 in, 2 out]
                  }
                }
                n239 = case shown="False" w225 {
                  tunnel: w224 -> [_ w240]
                  frame False {
                    n240 = local read "CtrlMode"() -> (w228:u32)
                    n241 = case shown="1, Default" w228 {
                      frame 1, Default {
                        w229 = u8 0 ("Disabled")
                        n242 = property on="I/E Range" class="Ring (strict)"("Disabled"=w229) -> ()  [unwired: 2 in, 2 out]
                        n243 = property on="I/E Autorange" class="Bool (strict)"("Disabled"=w229) -> ()  [unwired: 2 in, 2 out]
                      }
                      frame 0 {
                        w230 = u8 2 ("Disabled")
                        n244 = property on="I/E Range" class="Ring (strict)"("Disabled"=w230) -> ()  [unwired: 2 in, 2 out]
                        n245 = property on="I/E Autorange" class="Bool (strict)"("Disabled"=w230) -> ()  [unwired: 2 in, 2 out]
                      }
                    }
                  }
                  frame True {
                    w235 = u32 0 items=["Galvanostat", "Potentiostat", "ZRA"] ("CtrlMode")
                    n246 = invoke class="IGamryPstat" method="IERange"(reference=w240) -> ("IERange"=w238:i32)  [unwired: 2 in, 2 out]
                    n247 = local read "CtrlMode"() -> (w236:u32)
                    n248 = Equal?(x=w236, y=w235) -> (x = y?=w234:bool)
                    n249 = local read "First I/E Range"() -> (w237:i32)
                    n250 = Subtract(x=w238, y=w237) -> (x-y=w239:i32)
                    n251 = Select(t=2, s=w234, f=1) -> (s? t:f=w231:i32)
                    n252 = property on="I/E Range" class="Ring (strict)"("Value"=w239, "Disabled"=w231) -> ()  [unwired: 2 in, 2 out]
                  }
                }
              }
            }
            n253 = Equal?(x=w215, y="PC5") -> (x = y?=w218:bool)
            n254 = Equal?(x=w213, y=w214) -> (x = y?=w217:bool)
            n255 = And(x=w217, y=w218) -> (x .and. y?=w219:bool)
            n256 = Select(t=i32[] [0], s=w219, f=i32[] []) -> (s? t:f=w221:i32[])
            n257 = property on="CA Speed" class="Ring (strict)"("Disabled Items []"=w221) -> ()  [unwired: 2 in, 2 out]
          }
          event "Select Graph": Value Change {
            n258 = event-data() -> ("NewVal"=w249:u16)  [unwired: 1 in]
            n259 = case shown="1" w249 {
              frame 0, Default {
                n260 = property class="WFChart (strict)"("Visible"=TRUE) -> ()  [unwired: 2 in, 2 out]
                n261 = property on="I vs. V" class="XYGraph (strict)"("Visible"=FALSE) -> ()  [unwired: 2 in, 2 out]
              }
              frame 1 {
                n262 = property class="WFChart (strict)"("Visible"=FALSE) -> ()  [unwired: 2 in, 2 out]
                n263 = local write "XY Graph Flipped?"(FALSE ("XY Graph Flipped?")) -> ()
                n264 = local read "Taking Data"() -> (w252:bool)
                n265 = case shown="False" w252 {
                  frame False {
                    n266 = local read "Im History"() -> (w261:sgl[])
                    n267 = local read "Vf History"() -> (w262:sgl[])
                    n268 = Build Cluster Array(w262, w261) -> (w260:cluster{sgl, sgl}[])
                    n269 = local write "I vs. V"(w260) -> ()
                  }
                  frame True {
                  }
                }
                n270 = property on="I vs. V" class="XYGraph (strict)"("Visible"=TRUE, "X Scale.Name Label.Text"="Voltage (V)", "Y Scale.Name Label.Text"="Current (A)", "Transpose Array"=FALSE, "Plot.Plot Name"="I vs. V") -> ()  [unwired: 2 in, 2 out]
              }
              frame 2 {
                n271 = property class="WFChart (strict)"("Visible"=FALSE) -> ()  [unwired: 2 in, 2 out]
                n272 = local write "XY Graph Flipped?"(TRUE ("XY Graph Flipped?")) -> ()
                n273 = local read "Taking Data"() -> (w263:bool)
                n274 = case shown="False" w263 {
                  frame False {
                    n275 = local read "Im History"() -> (w272:sgl[])
                    n276 = local read "Vf History"() -> (w273:sgl[])
                    n277 = Build Cluster Array(w272, w273) -> (w271:cluster{sgl, sgl}[])
                    n278 = local write "I vs. V"(w271) -> ()
                  }
                  frame True {
                  }
                }
                n279 = property on="I vs. V" class="XYGraph (strict)"("Visible"=TRUE, "X Scale.Name Label.Text"="Current (A)", "Y Scale.Name Label.Text"="Voltage (V)", "Transpose Array"=FALSE, "Plot.Plot Name"="V vs. I") -> ()  [unwired: 2 in, 2 out]
              }
            }
          }
          event "Cell State": Value Change {
            n280 = event-data() -> ("NewVal"=w275:bool)  [unwired: 1 in, 5 out]
            n281 = local read "Device Open"() -> (w274:bool)
            n282 = case shown="True" w274 {
              tunnel: w275 -> [_ w278]
              frame False {
              }
              frame True {
                # "Monitor Cell Switch"
                n283 = Boolean To (0,1)(Boolean=w278) -> (0, 1=w279:i16)
                n284 = local read "Pstat"() -> (w280:refnum<k7>)
                n285 = invoke class="IGamryPstat" method="SetCell"(reference=w280, "CellState"=w279) -> ("SetCell"=w276:i32)  [unwired: 2 in, 3 out]
                n286 = Not Equal To 0?(x=w276) -> (x != 0?=→"SetCell":bool)
                "Cell Val Change NewVal" <- w278
              }
            }
          }
          event "CtrlMode", "I/E Range", "Vch Range", "Ich Range", "Vch Filter", "Ich Filter", "I/E Autorange", "Vch Autorange", "Ich Autorange", "Vch Offset", "Ich Offset", "VchOffsetEnable", "IchOffsetEnable", "ForcePstatFunctionUpdate", "I/E Stability", "CA Speed": Value Change {
            # "Adjust unit labels\naccording to\nControl Mode"
            n287 = event-data() -> ("CtlRef"=w282:refnum<vi>)  [unwired: 1 in]
            n288 = control-ref of="CtrlMode"() -> (w284:refnum<vi>)
            n289 = local write "ForcePstatFunctionUpdate"(FALSE ("ForcePstatFunctionUpdate")) -> ()
            n290 = To More Generic Class(target class=w282, reference=w284) -> (generic class reference=w283:refnum<vi>)
            n291 = local read "CtrlMode"() -> (w285:u32)
            n292 = Equal?(x=w282, y=w283) -> (x = y?=w286:bool)
            n293 = case shown="True" w286 {
              tunnel: w285 -> [_ w294]
              tunnel: [errorcluster {"status"=FALSE, "code"=0, "source"=""} ("error out") w293] -> w281
              frame False {
              }
              frame True {
                n294 = case shown="1, Default" w294 {
                  selector: w294 -> [_ w309]
                  tunnel: [w295 w314] -> w293
                  frame 0 {
                    w296 = u8 2 ("Disabled")
                    w298 = u16 0 items=["Fast", "Medium Fast", "Normal", "Slow"] ("I/E Stability")
                    w300 = "A" ("Caption.Text")
                    n295 = property on="Initial" class="DigNum (strict)"("Caption.Text"=w300) -> ()  [unwired: 2 in, 2 out]
                    n296 = property on="Amplitude" class="DigNum (strict)"("Caption.Text"=w300) -> ()  [unwired: 2 in, 2 out]
                    n297 = property on="DC Offset" class="DigNum (strict)"("Caption.Text"=w300) -> ()  [unwired: 2 in, 2 out]
                    n298 = property on="Final" class="DigNum (strict)"("Caption.Text"=w300) -> ()  [unwired: 2 in, 2 out]
                    n299 = property on="I/E Stability" class="Ring (strict)"("Disabled"=u8 2, "Value"=w298) -> ()  [unwired: 2 in, 2 out]
                    n300 = property on="Scan Rate" class="DigNum (strict)"("Caption.Text"="A/s") -> ()  [unwired: 2 in, 2 out]
                    n301 = property on="I/E Range" class="Ring (strict)"("Disabled"=w296) -> ()  [unwired: 2 in, 2 out]
                    n302 = property on="I/E Autorange" class="Bool (strict)"("Disabled"=w296, "Value"=TRUE) -> (error out=w295:errorcluster)  [unwired: 2 in, 1 out]
                  }
                  frame 1, Default {
                    w311 = u32 2 items=["Galvanostat", "Potentiostat", "ZRA"] ("CtrlMode")
                    w315 = u8 0 ("Disabled")
                    w317 = "V" ("Caption.Text")
                    n303 = local read "Family"() -> (w312:string)
                    n304 = Equal?(x=w309, y=w311) -> (x = y?=w310:bool)
                    n305 = property on="Initial" class="DigNum (strict)"("Caption.Text"=w317) -> ()  [unwired: 2 in, 2 out]
                    n306 = property on="Amplitude" class="DigNum (strict)"("Caption.Text"=w317) -> ()  [unwired: 2 in, 2 out]
                    n307 = property on="DC Offset" class="DigNum (strict)"("Caption.Text"=w317) -> ()  [unwired: 2 in, 2 out]
                    n308 = property on="Final" class="DigNum (strict)"("Caption.Text"=w317) -> ()  [unwired: 2 in, 2 out]
                    n309 = property on="I/E Stability" class="Ring (strict)"("Disabled"=u8 0) -> ()  [unwired: 2 in, 2 out]
                    n310 = property on="Scan Rate" class="DigNum (strict)"("Caption.Text"="V/s") -> ()  [unwired: 2 in, 2 out]
                    n311 = local read "CA Speed"() -> (w303:u16)
                    n312 = Equal?(x=w312, y="PC5") -> (x = y?=w308:bool)
                    n313 = Equal?(x=w303, y=u16 0) -> (x = y?=w306:bool)
                    n314 = Compound Arithmetic op=AND(w310, w308, w306) -> (w305:bool)
                    n315 = property on="I/E Range" class="Ring (strict)"("Disabled"=w315) -> ()  [unwired: 2 in, 2 out]
                    n316 = Select(t=u16 1, s=w305, f=w303) -> (s? t:f=w304:u16)
                    n317 = local write "CA Speed"(w304) -> ()
                    n318 = property on="I/E Autorange" class="Bool (strict)"("Disabled"=w315) -> (error out=w314:errorcluster)  [unwired: 2 in, 1 out]
                  }
                }
              }
            }
            n319 = local read "Device Open"() -> (w290:bool)
            n320 = local read "Pstat"() -> (w289:refnum<k7>)
            n321 = case shown="True" w290 {
              tunnel: w289 -> [_ w325]
              tunnel: [errorcluster {"status"=FALSE, "code"=0, "source"=""} ("error out") w332] -> w287
              tunnel: w281 -> [_ w321]
              frame False {
              }
              frame True {
                w364 = 0 items=["StabilityFast", "StabilityMedFast", "StabilityNorm", "StabilitySlow"] ("Stability")
                w367 = 0 items=["GstatMode", "PstatMode", "ZRAMode", "FRAMode"] ("SetCtrlMode")
                n322 = local read "CtrlMode"() -> (w385:u32)
                n323 = invoke class="IGamryPstat" method="SetCtrlMode"(reference=w325, error in=w321, "CtrlMode"=w385) -> (reference out=w361:refnum<k7>, error out=w362:errorcluster, "SetCtrlMode"=w366:i32)  [unwired: 1 in, 1 out]
                n324 = local read "IchOffsetEnable"() -> (w356:bool)
                n325 = local read "Ich Autorange"() -> (w374:bool)
                n326 = local read "Ich Range"() -> (w383:u16)
                n327 = local write "CtrlMode"(w366) -> ()
                n328 = invoke class="IGamryPstat" method="SetIchOffsetEnable"(reference=w325, "OffsetEnable"=w356) -> (reference out=w346:refnum<k7>, error out=w347:errorcluster, "SetIchOffsetEnable"=w357:bool)  [unwired: 2 in, 1 out]
                n329 = local read "VchOffsetEnable"() -> (w354:bool)
                n330 = invoke class="IGamryPstat" method="SetIchRangeMode"(reference=w325, "RangeMode"=w374) -> (reference out=w340:refnum<k7>, error out=w341:errorcluster, "SetIchRangeMode"=w375:bool)  [unwired: 2 in, 1 out]
                n331 = invoke class="IGamryPstat" method="SetIchRange"(reference=w325, "Range"=w383) -> (reference out=w344:refnum<k7>, error out=w345:errorcluster, "SetIchRange"=w384:i32)  [unwired: 2 in, 1 out]
                n332 = local read "Vch Autorange"() -> (w372:bool)
                n333 = local read "First I/E Range"() -> (w377:i32)
                n334 = Equal?(x=w366, y=w367) -> (x = y?=w368:bool)
                n335 = local read "I/E Stability"() -> (w365:u16)
                n336 = local read "Vch Range"() -> (w381:u16)
                n337 = local read "I/E Range"() -> (w376:u16)
                n338 = invoke class="IGamryPstat" method="SetVchOffsetEnable"(reference=w346, error in=w347, "OffsetEnable"=w354) -> (reference out=w324:refnum<k7>, error out=w323:errorcluster, "SetVchOffsetEnable"=w355:bool)  [unwired: 1 in, 1 out]
                n339 = local write "Ich Range"(w384) -> ()
                n340 = local write "IchOffsetEnable"(w357) -> ()
                n341 = local write "Ich Autorange"(w375) -> ()
                n342 = invoke class="IGamryPstat" method="SetVchRangeMode"(reference=w340, error in=w341, "RangeMode"=w372) -> (reference out=w338:refnum<k7>, error out=w339:errorcluster, "SetVchRangeMode"=w373:bool)  [unwired: 1 in, 1 out]
                n343 = invoke class="IGamryPstat" method="SetVchRange"(reference=w344, error in=w345, "Range"=w381) -> (reference out=w342:refnum<k7>, error out=w343:errorcluster, "SetVchRange"=w382:i32)  [unwired: 1 in, 1 out]
                n344 = local read "I/E Autorange"() -> (w370:bool)
                n345 = Select(t=w364, s=w368, f=w365) -> (s? t:f=w363:i32)
                n346 = Add(x=w376, y=w377) -> (x+y=w379:i32)
                n347 = local read "Ich Offset"() -> (w330:sgl)
                n348 = local read "Ich Filter"() -> (w352:u16)
                n349 = invoke class="IGamryPstat" method="SetIEStability"(reference=w361, error in=w362, "Stability"=w363) -> (reference out=w358:refnum<k7>, error out=w359:errorcluster, "SetIEStability"=w369:i32)  [unwired: 1 in, 1 out]
                n350 = invoke class="IGamryPstat" method="SetIchFilter"(reference=w325, "Filter"=w352) -> (reference out=w349:refnum<k7>, error out=w348:errorcluster, "SetIchFilter"=w353:i32)  [unwired: 2 in, 1 out]
                n351 = invoke class="IGamryPstat" method="SetIchOffset"(reference=w324, error in=w323, "Offset"=w330) -> (reference out=w327:refnum<k7>, error out=w326:errorcluster, "SetIchOffset"=w331:sgl)  [unwired: 1 in, 1 out]
                n352 = invoke class="IGamryPstat" method="SetIERange"(reference=w342, error in=w343, "Range"=w379) -> (error out=w334:errorcluster, "SetIERange"=w380:i32)  [unwired: 1 in, 2 out]
                n353 = local write "Vch Range"(w382) -> ()
                n354 = local write "VchOffsetEnable"(w355) -> ()
                n355 = invoke class="IGamryPstat" method="SetIERangeMode"(reference=w338, error in=w339, "RangeMode"=w370) -> (error out=w333:errorcluster, "SetIERangeMode"=w371:bool)  [unwired: 1 in, 2 out]
                n356 = local write "Vch Autorange"(w373) -> ()
                n357 = local read "Vch Offset"() -> (w329:sgl)
                n358 = local read "CA Speed"() -> (w320:u16)
                n359 = local read "Vch Filter"() -> (w351:u16)
                n360 = invoke class="IGamryPstat" method="SetCASpeed"(reference=w358, error in=w359, "CASpeed"=w320) -> (error out=w336:errorcluster, "SetCASpeed"=w360:i32)  [unwired: 1 in, 2 out]
                n361 = invoke class="IGamryPstat" method="SetVchFilter"(reference=w349, error in=w348, "Filter"=w351) -> (error out=w335:errorcluster, "SetVchFilter"=w350:i32)  [unwired: 1 in, 2 out]
                n362 = invoke class="IGamryPstat" method="SetVchOffset"(reference=w327, error in=w326, "Offset"=w329) -> (error out=w322:errorcluster, "SetVchOffset"=w328:sgl)  [unwired: 1 in, 2 out]
                n363 = local write "I/E Stability"(w369) -> ()
                n364 = local write "Ich Filter"(w353) -> ()
                n365 = local write "Ich Offset"(w331) -> ()
                n366 = local write "I/E Autorange"(w371) -> ()
                n367 = Subtract(x=w380, y=w377) -> (x-y=w378:i32)
                n368 = local write "CA Speed"(w360) -> ()
                n369 = local write "Vch Filter"(w350) -> ()
                n370 = local write "Vch Offset"(w328) -> ()
                n371 = local write "I/E Range"(w378) -> ()
                n372 = Build Array(w336, w335, w322, w334, w333) -> (w337:errorcluster[])
                n373 = Merge Errors(w337) -> (w332:errorcluster)
              }
            }
            n374 = Unbundle By Name(w287) -> ("status"=w288:bool)
            n375 = call "Pstat Settings Error"("Enable"=w288) -> ()  [unwired: 9 in, 2 out]
          }
          event "Cycles", "Signal Type", "Acq. Frequency", "Signal Frequency", "Amplitude", "DC Offset", "Phase Offset", "Initial", "Final", "Scan Rate", "Continuous", "Duty Cycle": Value Change {
            # "Signal Tweak Loop"
            n376 = event-data() -> ("OldVal"=w388:variant, "NewVal"=w387:variant, "CtlRef"=w386:refnum<vi>)  [unwired: 1 in]
            n377 = local read "Continuous"() -> (w389:bool)
            n378 = local read "Taking Data"() -> (w393:bool)
            n379 = local read "Signal Type"() -> (w394:u16)
            n380 = stacked-sequence {
              tunnel: w394 -> [w395 w426]
              tunnel: w393 -> [_ w425]
              tunnel: w388 -> [_ w424]
              tunnel: w387 -> [_ w423]
              tunnel: w386 -> [_ w422]
              frame #0 {
                # "Adjust front panel according to signal type"
                n381 = case shown="8" w395 {
                  frame 0, 1, 4 {
                    w397 = FALSE ("Visible")
                    (unwired) FALSE ("Visible")
                    w399 = TRUE ("Visible")
                    n382 = property on="Filename" class="Path"("Visible"=FALSE) -> ()  [unwired: 2 in, 2 out]
                    n383 = property on="Final" class="DigNum (strict)"("Visible"=w397) -> ()  [unwired: 2 in, 2 out]
                    n384 = property on="Initial" class="DigNum (strict)"("Visible"=w397) -> ()  [unwired: 2 in, 2 out]
                    n385 = property on="Scan Rate" class="DigNum (strict)"("Visible"=w397) -> ()  [unwired: 2 in, 2 out]
                    n386 = property on="Duty Cycle" class="DigNum (strict)"("Visible"=FALSE) -> ()  [unwired: 2 in, 2 out]
                    n387 = property on="DC Offset" class="DigNum (strict)"("Visible"=w399) -> ()  [unwired: 2 in, 2 out]
                    n388 = property on="Cycles" class="DigNum (strict)"("Visible"=w399) -> ()  [unwired: 2 in, 2 out]
                    n389 = property on="Signal Frequency" class="DigNum (strict)"("Visible"=w399) -> ()  [unwired: 2 in, 2 out]
                    n390 = property on="Amplitude" class="DigNum (strict)"("Visible"=w399) -> ()  [unwired: 2 in, 2 out]
                    n391 = property on="Phase Offset" class="DigNum (strict)"("Visible"=w399) -> ()  [unwired: 2 in, 2 out]
                    n392 = property on="Acq. Frequency" class="DigNum (strict)"("Visible"=w399) -> ()  [unwired: 2 in, 2 out]
                    n393 = property on="Continuous" class="Bool (strict)"("Visible"=w399) -> ()  [unwired: 2 in, 2 out]
                  }
                  frame 2 {
                    w401 = TRUE ("Visible")
                    (unwired) FALSE ("Visible")
                    w402 = FALSE ("Visible")
                    # "Triangle"
                    n394 = property on="Filename" class="Path"("Visible"=FALSE) -> ()  [unwired: 2 in, 2 out]
                    n395 = property on="Duty Cycle" class="DigNum (strict)"("Visible"=FALSE) -> ()  [unwired: 2 in, 2 out]
                    n396 = property on="Final" class="DigNum (strict)"("Visible"=w401) -> ()  [unwired: 2 in, 2 out]
                    n397 = property on="Initial" class="DigNum (strict)"("Visible"=w401) -> ()  [unwired: 2 in, 2 out]
                    n398 = property on="Scan Rate" class="DigNum (strict)"("Visible"=w401) -> ()  [unwired: 2 in, 2 out]
                    n399 = property on="Cycles" class="DigNum (strict)"("Visible"=w401) -> ()  [unwired: 2 in, 2 out]
                    n400 = property on="DC Offset" class="DigNum (strict)"("Visible"=w402) -> ()  [unwired: 2 in, 2 out]
                    n401 = property on="Continuous" class="Bool (strict)"("Visible"=w401) -> ()  [unwired: 2 in, 2 out]
                    n402 = property on="Acq. Frequency" class="DigNum (strict)"("Visible"=w401) -> ()  [unwired: 2 in, 2 out]
                    n403 = property on="Signal Frequency" class="DigNum (strict)"("Visible"=w402) -> ()  [unwired: 2 in, 2 out]
                    n404 = property on="Amplitude" class="DigNum (strict)"("Visible"=w402) -> ()  [unwired: 2 in, 2 out]
                    n405 = property on="Phase Offset" class="DigNum (strict)"("Visible"=w402) -> ()  [unwired: 2 in, 2 out]
                  }
                  frame 3 {
                    w406 = FALSE ("Visible")
                    (unwired) FALSE ("Visible")
                    w408 = TRUE ("Visible")
                    n406 = property on="Final" class="DigNum (strict)"("Visible"=w406) -> ()  [unwired: 2 in, 2 out]
                    n407 = property on="Initial" class="DigNum (strict)"("Visible"=w406) -> ()  [unwired: 2 in, 2 out]
                    n408 = property on="Scan Rate" class="DigNum (strict)"("Visible"=w406) -> ()  [unwired: 2 in, 2 out]
                    n409 = property on="Filename" class="Path"("Visible"=FALSE) -> ()  [unwired: 2 in, 2 out]
                    n410 = property on="Phase Offset" class="DigNum (strict)"("Visible"=FALSE) -> ()  [unwired: 2 in, 2 out]
                    n411 = property on="DC Offset" class="DigNum (strict)"("Visible"=w408) -> ()  [unwired: 2 in, 2 out]
                    n412 = property on="Cycles" class="DigNum (strict)"("Visible"=w408) -> ()  [unwired: 2 in, 2 out]
                    n413 = property on="Duty Cycle" class="DigNum (strict)"("Visible"=TRUE) -> ()  [unwired: 2 in, 2 out]
                    n414 = property on="Signal Frequency" class="DigNum (strict)"("Visible"=w408) -> ()  [unwired: 2 in, 2 out]
                    n415 = property on="Amplitude" class="DigNum (strict)"("Visible"=w408) -> ()  [unwired: 2 in, 2 out]
                    n416 = property on="Acq. Frequency" class="DigNum (strict)"("Visible"=w408) -> ()  [unwired: 2 in, 2 out]
                    n417 = property on="Continuous" class="Bool (strict)"("Visible"=w408) -> ()  [unwired: 2 in, 2 out]
                  }
                  frame 5, 6 {
                    w410 = TRUE ("Visible")
                    (unwired) FALSE ("Visible")
                    w411 = FALSE ("Visible")
                    # "Ramp"
                    n418 = property on="Filename" class="Path"("Visible"=FALSE) -> ()  [unwired: 2 in, 2 out]
                    n419 = property on="Duty Cycle" class="DigNum (strict)"("Visible"=FALSE) -> ()  [unwired: 2 in, 2 out]
                    n420 = property on="Final" class="DigNum (strict)"("Visible"=w410) -> ()  [unwired: 2 in, 2 out]
                    n421 = property on="Initial" class="DigNum (strict)"("Visible"=w410) -> ()  [unwired: 2 in, 2 out]
                    n422 = property on="Scan Rate" class="DigNum (strict)"("Visible"=w410) -> ()  [unwired: 2 in, 2 out]
                    n423 = property on="DC Offset" class="DigNum (strict)"("Visible"=w411) -> ()  [unwired: 2 in, 2 out]
                    n424 = property on="Cycles" class="DigNum (strict)"("Visible"=w411) -> ()  [unwired: 2 in, 2 out]
                    n425 = property on="Acq. Frequency" class="DigNum (strict)"("Visible"=w410) -> ()  [unwired: 2 in, 2 out]
                    n426 = property on="Signal Frequency" class="DigNum (strict)"("Visible"=w411) -> ()  [unwired: 2 in, 2 out]
                    n427 = property on="Amplitude" class="DigNum (strict)"("Visible"=w411) -> ()  [unwired: 2 in, 2 out]
                    n428 = property on="Phase Offset" class="DigNum (strict)"("Visible"=w411) -> ()  [unwired: 2 in, 2 out]
                    n429 = property on="Continuous" class="Bool (strict)"("Visible"=w411) -> ()  [unwired: 2 in, 2 out]
                  }
                  frame 7 {
                    w415 = FALSE ("Visible")
                    w413 = TRUE ("Visible")
                    w417 = FALSE ("Visible")
                    # "Single Point"
                    n430 = property on="Filename" class="Path"("Visible"=FALSE) -> ()  [unwired: 2 in, 2 out]
                    n431 = property on="Final" class="DigNum (strict)"("Visible"=w415) -> ()  [unwired: 2 in, 2 out]
                    n432 = property on="Initial" class="DigNum (strict)"("Visible"=w415) -> ()  [unwired: 2 in, 2 out]
                    n433 = property on="Scan Rate" class="DigNum (strict)"("Visible"=w415) -> ()  [unwired: 2 in, 2 out]
                    n434 = property on="Duty Cycle" class="DigNum (strict)"("Visible"=FALSE) -> ()  [unwired: 2 in, 2 out]
                    n435 = property on="DC Offset" class="DigNum (strict)"("Visible"=w413) -> ()  [unwired: 2 in, 2 out]
                    n436 = property on="Acq. Frequency" class="DigNum (strict)"("Visible"=w413) -> ()  [unwired: 2 in, 2 out]
                    n437 = property on="Cycles" class="DigNum (strict)"("Visible"=w417) -> ()  [unwired: 2 in, 2 out]
                    n438 = property on="Continuous" class="Bool (strict)"("Visible"=w417) -> ()  [unwired: 2 in, 2 out]
                    n439 = property on="Signal Frequency" class="DigNum (strict)"("Visible"=w417) -> ()  [unwired: 2 in, 2 out]
                    n440 = property on="Amplitude" class="DigNum (strict)"("Visible"=w417) -> ()  [unwired: 2 in, 2 out]
                    n441 = property on="Phase Offset" class="DigNum (strict)"("Visible"=w417) -> ()  [unwired: 2 in, 2 out]
                  }
                  frame 8 {
                    w419 = FALSE ("Visible")
                    w420 = TRUE ("Visible")
                    (unwired) FALSE ("Visible")
                    w421 = FALSE ("Visible")
                    # "From File"
                    n442 = property on="Final" class="DigNum (strict)"("Visible"=w419) -> ()  [unwired: 2 in, 2 out]
                    n443 = property on="Initial" class="DigNum (strict)"("Visible"=w419) -> ()  [unwired: 2 in, 2 out]
                    n444 = property on="Scan Rate" class="DigNum (strict)"("Visible"=w419) -> ()  [unwired: 2 in, 2 out]
                    n445 = property on="Duty Cycle" class="DigNum (strict)"("Visible"=FALSE) -> ()  [unwired: 2 in, 2 out]
                    n446 = property on="Filename" class="Path"("Visible"=w420) -> ()  [unwired: 2 in, 2 out]
                    n447 = property on="Cycles" class="DigNum (strict)"("Visible"=w420) -> ()  [unwired: 2 in, 2 out]
                    n448 = property on="DC Offset" class="DigNum (strict)"("Visible"=w421) -> ()  [unwired: 2 in, 2 out]
                    n449 = property on="Acq. Frequency" class="DigNum (strict)"("Visible"=w420) -> ()  [unwired: 2 in, 2 out]
                    n450 = property on="Continuous" class="Bool (strict)"("Visible"=w420) -> ()  [unwired: 2 in, 2 out]
                    n451 = property on="Signal Frequency" class="DigNum (strict)"("Visible"=w421) -> ()  [unwired: 2 in, 2 out]
                    n452 = property on="Amplitude" class="DigNum (strict)"("Visible"=w421) -> ()  [unwired: 2 in, 2 out]
                    n453 = property on="Phase Offset" class="DigNum (strict)"("Visible"=w421) -> ()  [unwired: 2 in, 2 out]
                  }
                  frame Default {
                  }
                }
              }
              frame #1 {
                n454 = case shown="True" w425 {
                  tunnel: w426 -> [_ w434]
                  tunnel: w424 -> [_ w429]
                  tunnel: w423 -> [_ w428]
                  tunnel: w422 -> [_ w427]
                  frame False {
                  }
                  frame True {
                    # "Nyquist Criterion"
                    n455 = local read "Signal Frequency"() -> (w430:dbl)
                    n456 = local read "Acq. Frequency"() -> (w431:dbl)
                    n457 = local read "Signal Type"() -> (w433:u16)
                    n458 = case shown="0, 1, 3, 4" w433 {
                      tunnel: w431 -> [_ w440]
                      tunnel: w430 -> [_ w438]
                      tunnel: [TRUE w436] -> w432
                      frame Default {
                      }
                      frame 0, 1, 3, 4 {
                        n459 = Multiply(x=2.0, y=w438) -> (x*y=w439:dbl)
                        n460 = Greater?(x=w440, y=w439) -> (0:w436:bool)
                      }
                    }
                    n461 = case shown="True" w432 {
                      tunnel: w430 -> [_ w464]
                      tunnel: w431 -> [_ w463]
                      tunnel: w434 -> [_ w460]
                      tunnel: w429 -> [_ w453]
                      tunnel: w428 -> [_ w452]
                      tunnel: w427 -> [_ w449]
                      frame False {
                        n462 = call "Nyquist Criterion"("Enable"=TRUE) -> ()  [unwired: 9 in, 2 out]
                      }
                      frame True {
                        w443 = 0 items=["SigTweakStyleReset", "SigTweakStyleContinue", "SigTweakStyleScale"] ("Tweak Style")
                        # "Check to see if the signal type changed,\nIf so, we want to RESET the tweak rather\nthan try and transition gracefully."
                        n463 = Not Equal?(x=w453, y=w452) -> (x != y?=w447:bool)
                        n464 = local read "Phase Offset"() -> (w467:dbl)
                        n465 = local read "Continuous"() -> (w461:bool)
                        n466 = local read "Amplitude"() -> (w465:dbl)
                        n467 = local read "Duty Cycle"() -> (w472:dbl)
                        n468 = local read "Scan Rate"() -> (w468:dbl)
                        n469 = local read "DC Offset"() -> (w466:dbl)
                        n470 = control-ref of="Signal Type"() -> (w451:refnum<vi>)
                        n471 = To More Generic Class(target class=w449, reference=w451) -> (generic class reference=w450:refnum<vi>)
                        n472 = local read "Cycles"() -> (w462:u32)
                        n473 = local read "Initial"() -> (w470:dbl)
                        n474 = local read "Final"() -> (w469:dbl)
                        n475 = case shown="7" w460 {
                          selector: w460 -> [w484 w500 w527 w542 _ _ _]
                          tunnel: w461 -> [w486 w502 w529 _ _ w575 w591]
                          tunnel: w462 -> [w485 w501 w528 _ _ w574 w590]
                          tunnel: w463 -> [w483 w499 w526 w550 w566 w573 w596]
                          tunnel: w464 -> [w475 _ w517 _ _ _ _]
                          tunnel: w465 -> [w482 _ w525 _ _ _ _]
                          tunnel: w466 -> [w481 _ w524 _ w560 _ _]
                          tunnel: w467 -> [w480 _ w523 _ _ _ _]
                          tunnel: w468 -> [_ w498 _ w549 _ _ _]
                          tunnel: w469 -> [_ w497 _ w548 _ _ _]
                          tunnel: w470 -> [_ w496 _ w547 _ _ _]
                          tunnel: [w479 w494 w522 w544 w564 w570 dbl[] []] -> w458
                          tunnel: [w478 w495 w521 1 ("t") -1 ("t") w571 w589] -> w459
                          tunnel: [w477 w493 w520 w545 w563 w572 w595] -> w455
                          tunnel: [w476 w492 w519 w543 0 ("error") 0 ("error") 0 ("error")] -> w471
                          tunnel: w472 -> [_ _ w518 _ _ _ _]
                          tunnel: [w473 w489 w515 w532 w561 w568 w588] -> w444
                          tunnel: w449 -> [_ _ _ w533 _ _ _]
                          frame 0, 1, 4 {
                            w473 = 2 items=["SigTweakStyleReset", "SigTweakStyleContinue", "SigTweakStyleScale"] ("Tweak Style")
                            # "Sine, Cosine, Sawtooth"
                            n476 = Select(t=-1, s=w486, f=w485) -> (s? t:f=w478:u32)
                            n477 = Reciprocal(x=w475) -> (1/x=w474:dbl)
                            n478 = Multiply(x=w483, y=w474) -> (x*y=w488:dbl)
                            n479 = call <vilib>:"Signal Generator by Duration.vi"("signal type"=w484, "duration"=w474, "# of samples"=w488, "frequency"=w475, "amplitude"=w482, "dc offset"=w481, "phase in"=w480) -> ("signal"=w479:dbl[], "error"=w476:i32)  [unwired: 5 in, 2 out]
                            n480 = Reciprocal(x=w483) -> (1/x=w477:dbl)
                          }
                          frame 2 {
                            w489 = 0 items=["SigTweakStyleReset", "SigTweakStyleContinue", "SigTweakStyleScale"] ("Tweak Style")
                            # "Triangle"
                            n481 = Add(x=w497, y=w496) -> (x+y=w503:dbl)
                            n482 = Subtract(x=w497, y=w496) -> (x-y=w507:dbl)
                            n483 = Select(t=-1, s=w502, f=w501) -> (s? t:f=w495:u32)
                            n484 = Divide(x=w507, y=w498) -> (x/y=w512:dbl)
                            n485 = Divide(x=w503, y=2.0) -> (x/y=w505:dbl)
                            n486 = Absolute Value(x=w512) -> (abs(x)=w511:dbl)
                            n487 = Divide(x=w507, y=2.0) -> (x/y=w506:dbl)
                            n488 = Multiply(x=w511, y=2.0) -> (x*y=w490:dbl)
                            n489 = Multiply(x=w499, y=w490) -> (x*y=w514:dbl)
                            n490 = Reciprocal(x=w490) -> (1/x=w491:dbl)
                            n491 = call <vilib>:"Signal Generator by Duration.vi"("signal type"=w500, "duration"=w490, "# of samples"=w514, "frequency"=w491, "amplitude"=w506, "dc offset"=w505, "phase in"=270.0) -> ("signal"=w494:dbl[], "error"=w492:i32)  [unwired: 5 in, 2 out]
                            n492 = Reciprocal(x=w499) -> (1/x=w493:dbl)
                          }
                          frame 3 {
                            w515 = 2 items=["SigTweakStyleReset", "SigTweakStyleContinue", "SigTweakStyleScale"] ("Tweak Style")
                            # "Square Wave"
                            n493 = Select(t=-1, s=w529, f=w528) -> (s? t:f=w521:u32)
                            n494 = Reciprocal(x=w517) -> (1/x=w516:dbl)
                            n495 = Multiply(x=w526, y=w516) -> (x*y=w531:dbl)
                            n496 = call <vilib>:"Signal Generator by Duration.vi"("signal type"=w527, "duration"=w516, "# of samples"=w531, "frequency"=w517, "amplitude"=w525, "dc offset"=w524, "phase in"=w523, "square wave duty cycle (%)"=w518) -> ("signal"=w522:dbl[], "error"=w519:i32)  [unwired: 4 in, 2 out]
                            n497 = Reciprocal(x=w526) -> (1/x=w520:dbl)
                          }
                          frame 5, 6 {
                            # "Ramp"
                            n498 = Subtract(x=w548, y=w547) -> (x-y=w552:dbl)
                            n499 = control-ref of="Scan Rate"() -> (w534:refnum<vi>)
                            n500 = control-ref of="Initial"() -> (w537:refnum<vi>)
                            n501 = Divide(x=w552, y=w549) -> (x/y=w551:dbl)
                            n502 = To More Generic Class(target class=w533, reference=w537) -> (generic class reference=w536:refnum<vi>)
                            n503 = To More Generic Class(target class=w533, reference=w534) -> (generic class reference=w535:refnum<vi>)
                            n504 = Equal?(x=w533, y=w536) -> (x = y?=w538:bool)
                            n505 = Equal?(x=w533, y=w535) -> (x = y?=w539:bool)
                            n506 = Absolute Value(x=w551) -> (abs(x)=w540:dbl)
                            n507 = case shown="False" w538 {
                              tunnel: w539 -> [w556 _]
                              tunnel: [w555 w559] -> w532
                              frame False {
                                n508 = case shown="False" w556 {
                                tunnel: [w557 w558] -> w555
                                frame False {
                                w557 = 1 items=["SigTweakStyleReset", "SigTweakStyleContinue", "SigTweakStyleScale"] ("Tweak Style")
                                }
                                frame True {
                                w558 = 2 items=["SigTweakStyleReset", "SigTweakStyleContinue", "SigTweakStyleScale"] ("Tweak Style")
                                }
                                }
                              }
                              frame True {
                                w559 = 0 items=["SigTweakStyleReset", "SigTweakStyleContinue", "SigTweakStyleScale"] ("Tweak Style")
                              }
                            }
                            n509 = Multiply(x=w550, y=w540) -> (x*y=w554:dbl)
                            n510 = Reciprocal(x=w540) -> (1/x=w541:dbl)
                            n511 = call <vilib>:"Signal Generator by Duration.vi"("signal type"=w542, "duration"=w540, "# of samples"=w554, "frequency"=w541, "amplitude"=w552, "dc offset"=w547, "phase in"=0.0) -> ("signal"=w544:dbl[], "error"=w543:i32)  [unwired: 5 in, 2 out]
                            n512 = Reciprocal(x=w550) -> (1/x=w545:dbl)
                          }
                          frame 7 {
                            w561 = 0 items=["SigTweakStyleReset", "SigTweakStyleContinue", "SigTweakStyleScale"] ("Tweak Style")
                            # "Single Point"
                            n513 = Reciprocal(x=w566) -> (1/x=w563:dbl)
                            n514 = Initialize Array(w560, 1 ("dimension size")) -> (w564:dbl[])
                          }
                          frame 8 {
                            w568 = 0 items=["SigTweakStyleReset", "SigTweakStyleContinue", "SigTweakStyleScale"] ("Tweak Style")
                            (unwired) TRUE ("convert eol (F)")
                            # "From File"
                            n515 = Select(t=-1, s=w575, f=w574) -> (s? t:f=w571:u32)
                            n516 = Reciprocal(x=w573) -> (1/x=w572:dbl)
                            n517 = local read "Filename"() -> (w586:path)
                            n518 = call <vilib>:"Open_Create_Replace File.vi"("file path"=w586) -> ("error out"=w583:errorcluster, "file size (bytes)"=w584:i32, "new file path"=w585:path, "refnum"=w587:refnum<file>)  [unwired: 7 in]
                            n519 = local write "Filename"(w585) -> ()
                            n520 = Read from Text File(file (use dialog)=w587, count=w584, error in=w583) -> (refnum out=w576:refnum<file>, text=w578:string, error out=w577:errorcluster)  [unwired: 1 in, 1 out]
                            n521 = Close File(refnum=w576, error in=w577) -> ()  [unwired: 2 out]
                            n522 = local write "From File Refnum"(w576) -> ()
                            n523 = local write "File Data"(w578) -> ()
                            n524 = Spreadsheet String To Array(delimiter (Tab)="\n", format string="%f", spreadsheet string=w578, array type (2D Dbl)=dbl[] [] ("initialized array")) -> (array=w570:dbl[])
                          }
                          frame Default {
                            w588 = 0 items=["SigTweakStyleReset", "SigTweakStyleContinue", "SigTweakStyleScale"] ("Tweak Style")
                            n525 = Select(t=-1, s=w591, f=w590) -> (s? t:f=w589:u32)
                            n526 = Reciprocal(x=w596) -> (1/x=w595:dbl)
                          }
                        }
                        n527 = Equal?(x=w449, y=w450) -> (x = y?=w446:bool)
                        n528 = And(x=w447, y=w446) -> (x .and. y?=w445:bool)
                        n529 = Select(t=w443, s=w445, f=w444) -> (s? t:f=w448:i32)
                        n530 = property class="WFChart (strict)"("X Scale.Offset and Multiplier:Multiplier"=w455) -> ()  [unwired: 2 in, 2 out]
                        n531 = call <vilib>:"Error Cluster From Error Code.vi"("error code (0)"=w471) -> ("error out"=w442:errorcluster)  [unwired: 8 in]
                        n532 = local read "Signal"() -> (w454:refnum<k7>)
                        n533 = call "SigArrayTweak.vi"("Signal IN"=w454, "Style"=w448, "Cycles"=w459, "Sample Rate"=w455, "Signal Array"=w458, "error in"=w442) -> ("error out"=w457:errorcluster)  [unwired: 8 in, 1 out]
                        n534 = Unbundle By Name(w457) -> ("status"=w456:bool)
                        n535 = call "Tweak Error"("Enable"=w456) -> ()  [unwired: 9 in, 2 out]
                      }
                    }
                  }
                }
              }
            }
            n536 = Select(t=2, s=w389, f=0) -> (s? t:f=w390:i32)
            n537 = property on="Cycles" class="DigNum (strict)"("Disabled"=w390) -> ()  [unwired: 2 in, 2 out]
          }
          event "Device List Change": Value Change {
            w608 = T2 0 items=["no dialog", "OK message", "continue or stop message", "OK message + warnings", "continue/stop + warnings"] ("type of dialog (OK msg:1)")
            n538 = event-data() -> ("CtlRef"=w598:refnum<vi>)  [unwired: 1 in, 5 out]
            n539 = property class="Bool (strict)"(reference=w598, "Value"=FALSE ("Device List Change")) -> ()  [unwired: 1 in, 2 out]
            n540 = local read "Section List"() -> (w605:string[])
            n541 = local read "Device List"() -> (w607:refnum<k7>)
            n542 = local read "Device"() -> (w606:u16)
            n543 = call "UpdateDeviceList.vi"("Section List"=w605, "Device"=w606, "Device List"=w607) -> ("error out"=w600:errorcluster, "New Section List"=w604:string[], "New Label List"=w602:string[], "New Device Index"=w601:i32)  [unwired: 5 in]
            n544 = local write "Index of Device (Device Change)"(w601) -> ()
            n545 = local write "Section List"(w604) -> ()
            n546 = Not Equal?(x=w601, y=-1) -> (x != y?=w611:bool)
            n547 = local read "Taking Data"() -> (w616:bool)
            n548 = Not(x=w611) -> (.not. x?=w610:bool)
            n549 = Select(t=w601, s=w611, f=0) -> (s? t:f=w612:i32)
            n550 = property on="Device" class="Ring (strict)"(error in=w600, "Strings []"=w602, "Value (Signaling)"=w612) -> (error out=w603:errorcluster)  [unwired: 1 in, 1 out]
            n551 = And(x=w610, y=w616) -> (x .and. y?=w615:bool)
            n552 = case shown="True" w615 {
              tunnel: w603 -> [w627 w629]
              tunnel: [w627 w629] -> w609
              frame False {
              }
              frame True {
                # "Stop and notify User"
                n553 = local write "Device Gone"(TRUE ("Device Gone")) -> ()
                n554 = local write "Start/Stop"(FALSE ("Start/Stop")) -> ()
                n555 = local write "Device Open"(FALSE ("Device Gone")) -> ()
              }
            }
            n556 = local read "[user-defined descriptions]"() -> (w618:string[])
            n557 = local read "[user-defined codes]"() -> (w617:u32[])
            n558 = local read "Taking Data"() -> (w599:bool)
            n559 = call <vilib>:"General Error Handler.vi"("[user-defined codes]"=w617, "[user-defined descriptions]"=w618, "type of dialog (OK msg:1)"=w608, "error in (no error)"=w609) -> ("error out"=w619:errorcluster)  [unwired: 7 in, 4 out]
            n560 = case shown="False" w599 {
              tunnel: w619 -> [w620 w624]
              frame False {
                n561 = case shown="No Error" w620 {
                  frame No Error {
                    w621 = u8 0 ("Disabled")
                    # "Enable appropriate menu stuff"
                    n562 = property on="Device" class="Ring (strict)"("Disabled"=w621) -> ()  [unwired: 2 in, 2 out]
                    n563 = property on="CtrlMode" class="Ring (strict)"("Disabled"=w621) -> ()  [unwired: 2 in, 2 out]
                    n564 = property on="I/E Range" class="Ring (strict)"("Disabled"=w621) -> ()  [unwired: 2 in, 2 out]
                    n565 = property on="Ich Range" class="Ring (strict)"("Disabled"=w621) -> ()  [unwired: 2 in, 2 out]
                    n566 = property on="Vch Filter" class="Ring (strict)"("Disabled"=w621) -> ()  [unwired: 2 in, 2 out]
                    n567 = property on="Ich Filter" class="Ring (strict)"("Disabled"=w621) -> ()  [unwired: 2 in, 2 out]
                    n568 = property on="Ich Offset" class="DigNum (strict)"("Disabled"=w621) -> ()  [unwired: 2 in, 2 out]
                    n569 = property on="CA Speed" class="Ring (strict)"("Disabled"=w621) -> ()  [unwired: 2 in, 2 out]
                    n570 = property on="Start/Stop" class="Bool (strict)"("Disabled"=w621) -> ()  [unwired: 2 in, 2 out]
                    n571 = property on="Signal Type" class="Ring (strict)"("Disabled"=w621) -> ()  [unwired: 2 in, 2 out]
                    n572 = property on="Vch Range" class="Ring (strict)"("Disabled"=w621) -> ()  [unwired: 2 in, 2 out]
                    n573 = property on="Vch Offset" class="DigNum (strict)"("Disabled"=w621) -> ()  [unwired: 2 in, 2 out]
                    n574 = property on="I/E Stability" class="Ring (strict)"("Disabled"=w621) -> ()  [unwired: 2 in, 2 out]
                  }
                  frame Error {
                    w623 = u16 0 items=[""] ("Device")
                    w622 = u8 2 ("Disabled")
                    # "Disable appropriate menu stuff"
                    n575 = property on="CtrlMode" class="Ring (strict)"("Disabled"=w622) -> ()  [unwired: 2 in, 2 out]
                    n576 = property on="Ich Offset" class="DigNum (strict)"("Disabled"=w622) -> ()  [unwired: 2 in, 2 out]
                    n577 = property on="CA Speed" class="Ring (strict)"("Disabled"=w622) -> ()  [unwired: 2 in, 2 out]
                    n578 = property on="Device" class="Ring (strict)"("Disabled"=w622, "Value"=w623) -> ()  [unwired: 2 in, 2 out]
                    n579 = property on="I/E Range" class="Ring (strict)"("Disabled"=w622, "Value"=w623) -> ()  [unwired: 2 in, 2 out]
                    n580 = property on="Ich Range" class="Ring (strict)"("Disabled"=w622, "Value"=w623) -> ()  [unwired: 2 in, 2 out]
                    n581 = property on="Vch Filter" class="Ring (strict)"("Disabled"=w622, "Value"=w623) -> ()  [unwired: 2 in, 2 out]
                    n582 = property on="Ich Filter" class="Ring (strict)"("Disabled"=w622, "Value"=w623) -> ()  [unwired: 2 in, 2 out]
                    n583 = property on="Start/Stop" class="Bool (strict)"("Disabled"=w622) -> ()  [unwired: 2 in, 2 out]
                    n584 = property on="Vch Offset" class="DigNum (strict)"("Disabled"=w622) -> ()  [unwired: 2 in, 2 out]
                    n585 = property on="I/E Stability" class="Ring (strict)"("Disabled"=w622) -> ()  [unwired: 2 in, 2 out]
                    n586 = property on="Vch Range" class="Ring (strict)"("Disabled"=w622, "Value"=w623) -> ()  [unwired: 2 in, 2 out]
                  }
                }
              }
              frame True {
                n587 = case shown="No Error" w624 {
                  frame No Error {
                  }
                  frame Error {
                    w626 = u16 0 items=[""] ("Device")
                    w625 = u8 2 ("Disabled")
                    # "Disable appropriate menu stuff"
                    n588 = property on="CtrlMode" class="Ring (strict)"("Disabled"=w625) -> ()  [unwired: 2 in, 2 out]
                    n589 = property on="Ich Offset" class="DigNum (strict)"("Disabled"=w625) -> ()  [unwired: 2 in, 2 out]
                    n590 = property on="CA Speed" class="Ring (strict)"("Disabled"=w625) -> ()  [unwired: 2 in, 2 out]
                    n591 = property on="Device" class="Ring (strict)"("Disabled"=w625, "Value"=w626) -> ()  [unwired: 2 in, 2 out]
                    n592 = property on="I/E Range" class="Ring (strict)"("Disabled"=w625, "Value"=w626) -> ()  [unwired: 2 in, 2 out]
                    n593 = property on="Ich Range" class="Ring (strict)"("Disabled"=w625, "Value"=w626) -> ()  [unwired: 2 in, 2 out]
                    n594 = property on="Vch Filter" class="Ring (strict)"("Disabled"=w625, "Value"=w626) -> ()  [unwired: 2 in, 2 out]
                    n595 = property on="Ich Filter" class="Ring (strict)"("Disabled"=w625, "Value"=w626) -> ()  [unwired: 2 in, 2 out]
                    n596 = property on="Start/Stop" class="Bool (strict)"("Disabled"=w625) -> ()  [unwired: 2 in, 2 out]
                    n597 = property on="Vch Offset" class="DigNum (strict)"("Disabled"=w625) -> ()  [unwired: 2 in, 2 out]
                    n598 = property on="I/E Stability" class="Ring (strict)"("Disabled"=w625) -> ()  [unwired: 2 in, 2 out]
                    n599 = property on="Vch Range" class="Ring (strict)"("Disabled"=w625, "Value"=w626) -> ()  [unwired: 2 in, 2 out]
                  }
                }
              }
            }
          }
          event "Device": Value Change {
            n600 = event-data() -> ("NewVal"=w633:u16)  [unwired: 1 in, 5 out]
            n601 = local read "Section List"() -> (w634:string[])
            n602 = Index Array(array=w634, index=w633) -> (element=w632:string)
            n603 = property on="Section" class="Str"("Value (Signaling)"=w632) -> ()  [unwired: 2 in, 2 out]
          }
          event "Section": Value Change {
            n604 = event-data() -> ("OldVal"=w636:string, "NewVal"=w635:string)  [unwired: 1 in, 4 out]
            n605 = Not Equal?(x=w636, y=w635) -> (x != y?=w637:bool)
            n606 = case shown="True" w637 {
              tunnel: w635 -> [_ w644]
              frame False {
              }
              frame True {
                n607 = local read "Device Open"() -> (w649:bool)
                n608 = local read "Pstat"() -> (w651:refnum<k7>)
                n609 = case shown="True" w649 {
                  tunnel: w651 -> [w696 w700]
                  tunnel: [w696 w699] -> w650
                  tunnel: [errorcluster {"status"=FALSE, "code"=0, "source"=""} ("error out") w697] -> w648
                  frame False {
                  }
                  frame True {
                    n610 = invoke class="IGamryPstat" method="Close"(reference=w700, "Safe"=TRUE) -> (reference out=w699:refnum<k7>, error out=w697:errorcluster)  [unwired: 2 in, 2 out]
                  }
                }
                n611 = invoke class="IGamryPstat" method="Init"(reference=w650, error in=w648, "Section"=w644) -> (reference out=w647:refnum<k7>, error out=w646:errorcluster)  [unwired: 1 in, 2 out]
                n612 = invoke class="IGamryPstat" method="Open"(reference=w647, error in=w646) -> (reference out=w640:refnum<k7>, error out=w645:errorcluster)  [unwired: 1 in, 1 out]
                n613 = case shown="No Error" w645 {
                  selector: w645 -> [w691 w693]
                  tunnel: [w691 w693] -> w641
                  frame No Error {
                    n614 = local write "Device Open"(TRUE ("Device Open")) -> ()
                  }
                  frame Error {
                    n615 = local write "Device Open"(FALSE ("Device Open")) -> ()
                  }
                }
                n616 = call "HardwareRangeStrings.vi"("error in (no error)"=w641, "Pstat IN"=w640) -> ("error out"=w642:errorcluster, "Hardware Strings"=w638:T10, "Pstat OUT"=w639:refnum<k7>)  [unwired: 7 in]
                n617 = invoke class="IGamryPstat" method="CtrlMode"(reference=w639, error in=w642) -> (reference out=w677:refnum<k7>, error out=w678:errorcluster, "CtrlMode"=w686:i32)  [unwired: 1 in]
                n618 = Unbundle By Name(w638) -> ("I/E Ranges"=w683:string[], "First I/E Range"=w671:i32, "VchRanges"=w685:string[], "IchRanges"=w684:string[], "VchFilters"=w682:string[], "IchFilters"=w681:string[], "Family"=w643:string, "CA Speeds"=w674:string[])  [unwired: 2 out]
                n619 = property on="I/E Range" class="Ring (strict)"("Strings []"=w683) -> ()  [unwired: 2 in, 2 out]
                n620 = local write "CtrlMode"(w686) -> ()
                n621 = property on="Ich Range" class="Ring (strict)"("Strings []"=w684) -> ()  [unwired: 2 in, 2 out]
                n622 = property on="Vch Filter" class="Ring (strict)"("Strings []"=w682) -> ()  [unwired: 2 in, 2 out]
                n623 = property on="Ich Filter" class="Ring (strict)"("Strings []"=w681) -> ()  [unwired: 2 in, 2 out]
                n624 = local write "Family"(w643) -> ()
                n625 = property on="CA Speed" class="Ring (strict)"("Strings []"=w674) -> ()  [unwired: 2 in, 2 out]
                n626 = invoke class="IGamryPstat" method="IchRange"(reference=w677, error in=w678) -> (reference out=w675:refnum<k7>, error out=w676:errorcluster, "IchRange"=w688:i32)  [unwired: 1 in]
                n627 = local write "Ich Range"(w688) -> ()
                n628 = property on="Vch Range" class="Ring (strict)"("Strings []"=w685) -> ()  [unwired: 2 in, 2 out]
                n629 = local write "First I/E Range"(w671) -> ()
                n630 = invoke class="IGamryPstat" method="VchRange"(reference=w675, error in=w676) -> (reference out=w658:refnum<k7>, error out=w659:errorcluster, "VchRange"=w687:i32)  [unwired: 1 in]
                n631 = local write "Vch Range"(w687) -> ()
                n632 = invoke class="IGamryPstat" method="IchFilter"(reference=w658, error in=w659) -> (reference out=w664:refnum<k7>, error out=w665:errorcluster, "IchFilter"=w663:i32)  [unwired: 1 in]
                n633 = local write "Ich Filter"(w663) -> ()
                n634 = invoke class="IGamryPstat" method="VchFilter"(reference=w664, error in=w665) -> (reference out=w656:refnum<k7>, error out=w657:errorcluster, "VchFilter"=w662:i32)  [unwired: 1 in]
                n635 = local write "Vch Filter"(w662) -> ()
                n636 = invoke class="IGamryPstat" method="IchOffset"(reference=w656, error in=w657) -> (reference out=w667:refnum<k7>, error out=w666:errorcluster, "IchOffset"=w661:sgl)  [unwired: 1 in]
                n637 = local write "Ich Offset"(w661) -> ()
                n638 = invoke class="IGamryPstat" method="VchOffset"(reference=w667, error in=w666) -> (reference out=w654:refnum<k7>, error out=w655:errorcluster, "VchOffset"=w660:sgl)  [unwired: 1 in]
                n639 = local write "Vch Offset"(w660) -> ()
                n640 = invoke class="IGamryPstat" method="CASpeed"(reference=w654, error in=w655) -> (reference out=w673:refnum<k7>, error out=w672:errorcluster, "CASpeed"=w669:i32)  [unwired: 1 in]
                n641 = invoke class="IGamryPstat" method="IEStability"(reference=w673, error in=w672) -> (reference out=w652:refnum<k7>, error out=w653:errorcluster, "IEStability"=w670:i32)  [unwired: 1 in]
                n642 = local write "CA Speed"(w669) -> ()
                n643 = local read "[user-defined descriptions]"() -> (w679:string[])
                n644 = local read "[user-defined codes]"() -> (w680:u32[])
                n645 = invoke class="IGamryPstat" method="IERange"(reference=w652, error in=w653) -> (error out=w668:errorcluster, "IERange"=w689:i32)  [unwired: 1 in, 1 out]
                n646 = local write "I/E Stability"(w670) -> ()
                n647 = call <vilib>:"General Error Handler.vi"("[user-defined codes]"=w680, "[user-defined descriptions]"=w679, "error in (no error)"=w668) -> ()  [unwired: 8 in, 5 out]
                n648 = Subtract(x=w689, y=w671) -> (x-y=w690:i32)
                n649 = local write "I/E Range"(w690) -> ()
              }
            }
          }
        }
      }
      n650 = while {
        stop <- w702 continue-if-true
        n651 = local read "Close"() -> (w703:bool)
        n652 = local read "milliseconds to wait"() -> (w701:u32)
        n653 = Not(x=w703) -> (.not. x?=w702:bool)
        n654 = event shown="[0] \"Start/Stop\": Value Change" {
          selector: _ -> [_ _]
          dyn-events: _ -> [_ _]
          timeout: w701 -> [_ _]
          event "Start/Stop": Value Change {
            n655 = event-data() -> ("NewVal"=w704:bool)  [unwired: 1 in, 4 out]
            n656 = case shown="True" w704 {
              frame False {
              }
              frame True {
                n657 = while {
                  shift-right: [w709] -> _
                  shift-left: DataAcqStates."Initialize" ("Data Acq States") -> [w712]
                  shift-right: [w707] -> _
                  shift-left: errorcluster {"status"=FALSE, "code"=0, "source"=""} ("error in (no error)") -> [w708]
                  stop <- w713 stop-if-true
                  n658 = case shown="\"Acquire Data\"" w712 {
                    tunnel: [DataAcqStates."Initialize Objects" ("Data Acq States") w779 w794 w986 w1002 w1166 DataAcqStates."STOP" ("Data Acq States")] -> w709
                    tunnel: w708 -> [w718 w759 w795 w987 w1003 w1168 w1204]
                    tunnel: [w718 w769 w793 w984 w1001 w1165 w1195] -> w707
                    frame "Initialize", Default {
                      w714 = u8 2 ("Disabled")
                      w716 = path "" ("Log File")
                      w717 = sgl[] [] ("Vf History")
                      w715 = FALSE
                      # "Disable appropriate menu items"
                      # "Initalize Chart and Lists"
                      n659 = local write "Vf History"(w717) -> ()
                      n660 = local write "Im History"(w717) -> ()
                      n661 = property on="CtrlMode" class="Ring (strict)"("Disabled"=w714) -> ()  [unwired: 2 in, 2 out]
                      n662 = property on="Log File" class="Path"("Value"=w716) -> ()  [unwired: 2 in, 2 out]
                      n663 = property class="WFChart (strict)"("History Data"=sgl[][] []) -> ()  [unwired: 2 in, 2 out]
                      n664 = property on="I vs. V" class="XYGraph (strict)"("Value"=cluster{dbl, dbl}[] [] ("I vs. V")) -> ()  [unwired: 2 in, 2 out]
                      n665 = local write "Current Overload"(w715) -> ()
                      n666 = local write "Control Amp Overload"(w715) -> ()
                      n667 = local write "Voltage Overload"(w715) -> ()
                      n668 = local read "Legacy Save"() -> (w720:bool)
                      n669 = local read "Continuous"() -> (w724:bool)
                      n670 = property on="Device" class="Ring (strict)"("Disabled"=w714) -> ()  [unwired: 2 in, 2 out]
                      n671 = property on="Acq. Frequency" class="DigNum (strict)"("Disabled"=w714) -> ()  [unwired: 2 in, 2 out]
                      n672 = property on="Legacy Save" class="Bool (strict)"("Disabled"=w714) -> ()  [unwired: 2 in, 2 out]
                      n673 = case shown="True" w720 {
                        tunnel: [FALSE w755] -> w719
                        tunnel: w716 -> [_ _]
                        frame False {
                          n674 = local read "Front Panel Window:Title"() -> (w729:string)
                          n675 = property class="VI"("Front Panel Window:Title"=w729) -> ()  [unwired: 2 in, 2 out]
                        }
                        frame True {
                          (unwired) T11."new or existing file" ("select mode (2)")
                          n676 = call <vilib>:"Open Registry Key.vi"("security access mask (KEY_READ | KEY_WRITE)"=Registry_SAM."KEY_READ", "subkey"="SOFTWARE\\Microsoft\\Windows\\CurrentVersion\\Explorer\\Shell Folders\\", "root key (HKEY_LOCAL_MACHINE)"=Registry_RtKey."HKEY_LOCAL_MACHINE") -> ("error out"=w736:errorcluster, "refnum out"=w738:T12)  [unwired: 7 in]
                          n677 = call-poly <vilib>:"Read Registry Value Simple.vi"("error in (no error)"=w736, "default data"="C:\\Documents and Settings\\All Users\\Documents\\", "value"="Common Documents", "refnum"=w738) -> ("error out"=w737:errorcluster, "String/Binary data"=w744:string, "refnum out"=w739:T12)  [unwired: 2 in, 1 out]
                          n678 = call <vilib>:"Close Registry Key.vi"("error in (no error)"=w737, "refnum"=w739) -> ()  [unwired: 5 in, 1 out]
                          n679 = Concatenate Strings(w744, "\\My Gamry Data\\" ("string")) -> (w746:string)
                          n680 = String To Path(string=w746) -> (path=w734:path)
                          n681 = File Dialog(6:"*.txt" ("pattern"), 7:"Data File Location" ("prompt"), 9:"logfile.txt" ("default name"), 11:w734) -> (0:w731:errorcluster, 3:w732:path)  [unwired: 3 in, 2 out]
                          n682 = Unbundle(w731) -> ()  [unwired: 3 out]
                          n683 = local read "Front Panel Window:Title"() -> (w751:string)
                          n684 = local write "Log File"(w732) -> ()
                          n685 = Path To String(path=w732) -> (string=w749:string)
                          n686 = call <vilib>:"Open_Create_Replace File.vi"("function (open:0)"=T8."create or replace", "file path"=w732) -> ("error out"=w756:errorcluster, "refnum"=w758:refnum<file>)  [unwired: 6 in, 2 out]
                          n687 = local write "Log File Refnum"(w758) -> ()
                          n688 = Unbundle By Name(w756) -> ("status"=w753:bool)
                          n689 = Empty String/Path?(string/path=w732) -> (empty?=w754:bool)
                          n690 = Or(x=w754, y=w753) -> (x .or. y?=w755:bool)
                          n691 = Concatenate Strings(w751, " - " ("string"), w749) -> (w752:string)
                          n692 = property class="VI"("Front Panel Window:Title"=w752) -> ()  [unwired: 2 in, 2 out]
                        }
                      }
                      n693 = Select(t=2, s=w724, f=0) -> (s? t:f=w723:i32)
                      n694 = property on="Cycles" class="DigNum (strict)"("Disabled"=w723) -> ()  [unwired: 2 in, 2 out]
                      n695 = call "Log File Error"("Enable"=w719) -> ()  [unwired: 9 in, 2 out]
                      n696 = case shown="True" w719 {
                        frame False {
                        }
                        frame True {
                          n697 = local write "Legacy Save"(FALSE) -> ()
                        }
                      }
                    }
                    frame "Initialize Objects" {
                      # "Register a sub VI to handle our DataAvailable and DataDone events"
                      n698 = local read "Pstat"() -> (w760:refnum<k7>)
                      n699 = invoke class="IGamryPstat" method="ModelNo"(reference=w760, error in=w759) -> (reference out=w761:refnum<k7>, error out=w762:errorcluster, "ModelNo"=w765:i32)  [unwired: 1 in]
                      n700 = Equal?(x=w765, y=4) -> (x = y?=w763:bool)
                      n701 = case shown="True" w763 {
                        tunnel: w761 -> [w781 w786]
                        tunnel: w762 -> [w780 w785]
                        tunnel: [w781 w784] -> w767
                        tunnel: [w780 w783] -> w766
                        frame False {
                        }
                        frame True {
                          n702 = invoke class="IGamryPstat" method="SetExtSrceEnable"(reference=w786, error in=w785, "ExtSrceEnable"=TRUE) -> (reference out=w784:refnum<k7>, error out=w783:errorcluster)  [unwired: 1 in, 2 out]
                        }
                      }
                      n703 = local read "CtrlMode"() -> (w772:u32)
                      n704 = invoke class="IGamryPstat" method="SetCtrlMode"(reference=w767, error in=w766, "CtrlMode"=w772) -> (reference out=w774:refnum<k7>, error out=w773:errorcluster, "SetCtrlMode"=w770:i32)  [unwired: 1 in, 1 out]
                      n705 = local write "CtrlMode"(w770) -> ()
                      n706 = local read "Dtaq"() -> (w771:refnum<k7>)
                      n707 = invoke class="IGamryDtaqIv" method="Init"(reference=w771, error in=w773, "Pstat"=w774) -> (reference out=w778:refnum<k7>, error out=w777:errorcluster)  [unwired: 1 in, 2 out]
                      n708 = control-ref of="DataDone?"() -> (w775:refnum<vi>)
                      n709 = vi-ref "DtaqDataDoneCallback - DtaqIV.vi"() -> ("vi reference"=w768:refnum<vi>)
                      n710 = node(w777, w778, w768, w775) -> (w776:refnum<k27>, w769:errorcluster)  [unwired: 1 in]
                      n711 = local write "DataDone Callback"(w776) -> ()
                      n712 = case shown="No Error" w769 {
                        tunnel: [DataAcqStates."Generate Signal" ("Data Acq States") DataAcqStates."STOP" ("Data Acq States")] -> w779
                        frame No Error {
                        }
                        frame Error {
                        }
                      }
                    }
                    frame "Generate Signal" {
                      # "Nyquist Criterion"
                      n713 = local read "Signal Frequency"() -> (w791:dbl)
                      n714 = local read "Acq. Frequency"() -> (w792:dbl)
                      n715 = local read "Signal Type"() -> (w789:u16)
                      n716 = case shown="0, 1, 3, 4" w789 {
                        tunnel: w792 -> [_ w801]
                        tunnel: w791 -> [_ w799]
                        tunnel: [TRUE w797] -> w790
                        frame Default {
                        }
                        frame 0, 1, 3, 4 {
                          n717 = Multiply(x=2.0, y=w799) -> (x*y=w800:dbl)
                          n718 = Greater?(x=w801, y=w800) -> (0:w797:bool)
                        }
                      }
                      n719 = case shown="True" w790 {
                        tunnel: w791 -> [_ w825]
                        tunnel: w792 -> [_ w809]
                        tunnel: w795 -> [w803 w817]
                        tunnel: [DataAcqStates."STOP" ("Data Acq States") w815] -> w794
                        tunnel: [w802 w806] -> w793
                        frame False {
                          n720 = call "Nyquist Criterion"("error in (no error)"=w803, "Enable"=TRUE) -> ("error out"=w802:errorcluster)  [unwired: 8 in, 1 out]
                        }
                        frame True {
                          n721 = local read "Phase Offset"() -> (w828:dbl)
                          n722 = local read "Signal Type"() -> (w822:u16)
                          n723 = local read "Continuous"() -> (w823:bool)
                          n724 = local read "Duty Cycle"() -> (w839:dbl)
                          n725 = local read "Amplitude"() -> (w826:dbl)
                          n726 = local read "Scan Rate"() -> (w829:dbl)
                          n727 = local read "DC Offset"() -> (w827:dbl)
                          n728 = local read "Cycles"() -> (w824:u32)
                          n729 = local read "Initial"() -> (w831:dbl)
                          n730 = local read "Final"() -> (w830:dbl)
                          n731 = case shown="2" w822 {
                            selector: w822 -> [w865 w872 w907 w917 _ _ w960 _]
                            tunnel: w823 -> [w867 w882 w909 _ _ w947 _ w978]
                            tunnel: w824 -> [w866 w881 w908 _ _ w946 _ w977]
                            tunnel: w809 -> [w856 w880 w906 w914 w934 w945 w961 w983]
                            tunnel: w825 -> [w855 _ w897 _ _ _ _ _]
                            tunnel: w826 -> [w864 _ w905 _ _ _ _ _]
                            tunnel: w827 -> [w863 _ w904 _ w929 _ _ _]
                            tunnel: w828 -> [w862 _ w903 _ _ _ _ _]
                            tunnel: w829 -> [_ w879 _ w923 _ _ w962 _]
                            tunnel: w830 -> [_ w878 _ w922 _ _ w963 _]
                            tunnel: w831 -> [_ w877 _ w921 _ _ w964 _]
                            tunnel: [w861 w875 w902 w919 w932 w942 w966 dbl[] []] -> w832
                            tunnel: [w860 w876 w901 1 ("t") -1 ("t") w943 1 ("t") w976] -> w842
                            tunnel: [w859 w874 w900 w915 w931 w944 w967 w982] -> w811
                            tunnel: [w858 w873 w899 w918 0 ("error") 0 ("error") w965 0 ("error")] -> w838
                            tunnel: w839 -> [_ _ w898 _ _ _ _ _]
                            frame 0, 1, 4 {
                              # "Sine, Cosine, Sawtooth"
                              n732 = Select(t=-1, s=w867, f=w866) -> (s? t:f=w860:u32)
                              n733 = Reciprocal(x=w855) -> (1/x=w854:dbl)
                              n734 = local write "Recording IV"(FALSE) -> ()
                              n735 = Multiply(x=w856, y=w854) -> (x*y=w857:dbl)
                              n736 = call <vilib>:"Signal Generator by Duration.vi"("signal type"=w865, "duration"=w854, "# of samples"=w857, "frequency"=w855, "amplitude"=w864, "dc offset"=w863, "phase in"=w862) -> ("signal"=w861:dbl[], "error"=w858:i32)  [unwired: 5 in, 2 out]
                              n737 = Reciprocal(x=w856) -> (1/x=w859:dbl)
                            }
                            frame 2 {
                              # "Triangle"
                              n738 = Add(x=w878, y=w877) -> (x+y=w883:dbl)
                              n739 = Subtract(x=w878, y=w877) -> (x-y=w887:dbl)
                              n740 = Select(t=-1, s=w882, f=w881) -> (s? t:f=w876:u32)
                              n741 = local write "Recording IV"(FALSE) -> ()
                              n742 = Divide(x=w887, y=w879) -> (x/y=w892:dbl)
                              n743 = Divide(x=w883, y=2.0) -> (x/y=w885:dbl)
                              n744 = Absolute Value(x=w892) -> (abs(x)=w891:dbl)
                              n745 = Divide(x=w887, y=2.0) -> (x/y=w886:dbl)
                              n746 = Multiply(x=w891, y=2.0) -> (x*y=w870:dbl)
                              n747 = Multiply(x=w880, y=w870) -> (x*y=w894:dbl)
                              n748 = Reciprocal(x=w870) -> (1/x=w871:dbl)
                              n749 = call <vilib>:"Signal Generator by Duration.vi"("signal type"=w872, "duration"=w870, "# of samples"=w894, "frequency"=w871, "amplitude"=w886, "dc offset"=w885, "phase in"=270.0) -> ("signal"=w875:dbl[], "error"=w873:i32)  [unwired: 5 in, 2 out]
                              n750 = Reciprocal(x=w880) -> (1/x=w874:dbl)
                            }
                            frame 3 {
                              # "Square Wave"
                              n751 = Select(t=-1, s=w909, f=w908) -> (s? t:f=w901:u32)
                              n752 = Reciprocal(x=w897) -> (1/x=w896:dbl)
                              n753 = local write "Recording IV"(FALSE) -> ()
                              n754 = Multiply(x=w906, y=w896) -> (x*y=w911:dbl)
                              n755 = call <vilib>:"Signal Generator by Duration.vi"("signal type"=w907, "duration"=w896, "# of samples"=w911, "frequency"=w897, "amplitude"=w905, "dc offset"=w904, "phase in"=w903, "square wave duty cycle (%)"=w898) -> ("signal"=w902:dbl[], "error"=w899:i32)  [unwired: 4 in, 2 out]
                              n756 = Reciprocal(x=w906) -> (1/x=w900:dbl)
                            }
                            frame 5, 6 {
                              # "Ramp"
                              n757 = Subtract(x=w922, y=w921) -> (x-y=w925:dbl)
                              n758 = local write "Recording IV"(TRUE) -> ()
                              n759 = Divide(x=w925, y=w923) -> (x/y=w924:dbl)
                              n760 = Absolute Value(x=w924) -> (abs(x)=w913:dbl)
                              n761 = Multiply(x=w914, y=w913) -> (x*y=w927:dbl)
                              n762 = Reciprocal(x=w913) -> (1/x=w916:dbl)
                              n763 = call <vilib>:"Signal Generator by Duration.vi"("signal type"=w917, "duration"=w913, "# of samples"=w927, "frequency"=w916, "amplitude"=w925, "dc offset"=w921, "phase in"=0.0) -> ("signal"=w919:dbl[], "error"=w918:i32)  [unwired: 5 in, 2 out]
                              n764 = Reciprocal(x=w914) -> (1/x=w915:dbl)
                            }
                            frame 7 {
                              # "Single Point"
                              n765 = local write "Recording IV"(FALSE) -> ()
                              n766 = Reciprocal(x=w934) -> (1/x=w931:dbl)
                              n767 = Initialize Array(w929, 1 ("dimension size")) -> (w932:dbl[])
                            }
                            frame 8 {
                              w939 = T13 2 items=["both", "start of string", "end of string"] ("location (both)")
                              (unwired) TRUE ("convert eol (F)")
                              # "From File"
                              n768 = local write "Recording IV"(FALSE) -> ()
                              n769 = Select(t=-1, s=w947, f=w946) -> (s? t:f=w943:u32)
                              n770 = local read "Filename"() -> (w957:path)
                              n771 = Reciprocal(x=w945) -> (1/x=w944:dbl)
                              n772 = call <vilib>:"Open_Create_Replace File.vi"("function (open:0)"=T8."open (read only)", "file path"=w957) -> ("error out"=w954:errorcluster, "file size (bytes)"=w955:i32, "new file path"=w956:path, "refnum"=w958:refnum<file>)  [unwired: 6 in]
                              n773 = local write "Filename"(w956) -> ()
                              n774 = Read from Text File(file (use dialog)=w958, count=w955, error in=w954) -> (refnum out=w948:refnum<file>, text=w938:string, error out=w949:errorcluster)  [unwired: 1 in, 1 out]
                              n775 = Close File(refnum=w948, error in=w949) -> ()  [unwired: 2 out]
                              n776 = local write "From File Refnum"(w948) -> ()
                              n777 = call <vilib>:"Trim Whitespace.vi"("string"=w938, "location (both)"=w939) -> ("trimmed string"=w937:string)
                              n778 = local write "File Data"(w937) -> ()
                              n779 = Spreadsheet String To Array(delimiter (Tab)="\n", format string="%f", spreadsheet string=w937, array type (2D Dbl)=dbl[] [] ("initialized array")) -> (array=w942:dbl[])
                            }
                            frame 9 {
                              # "IV Curve"
                              n780 = Subtract(x=w963, y=w964) -> (x-y=w972:dbl)
                              n781 = local write "Recording IV"(TRUE) -> ()
                              n782 = Divide(x=w972, y=w962) -> (x/y=w971:dbl)
                              n783 = Absolute Value(x=w971) -> (abs(x)=w969:dbl)
                              n784 = Multiply(x=w961, y=w969) -> (x*y=w974:dbl)
                              n785 = Reciprocal(x=w969) -> (1/x=w970:dbl)
                              n786 = call <vilib>:"Signal Generator by Duration.vi"("signal type"=w960, "duration"=w969, "# of samples"=w974, "frequency"=w970, "amplitude"=w972, "dc offset"=w964, "phase in"=0.0) -> ("signal"=w966:dbl[], "error"=w965:i32)  [unwired: 5 in, 2 out]
                              n787 = Reciprocal(x=w961) -> (1/x=w967:dbl)
                            }
                            frame Default {
                              n788 = Select(t=-1, s=w978, f=w977) -> (s? t:f=w976:u32)
                              n789 = local write "Recording IV"(FALSE) -> ()
                              n790 = Reciprocal(x=w983) -> (1/x=w982:dbl)
                            }
                          }
                          n791 = local read "Log File Refnum"() -> (w841:refnum<file>)
                          n792 = local read "Legacy Save"() -> (w840:bool)
                          n793 = local read "CtrlMode"() -> (w814:u32)
                          n794 = call <vilib>:"Error Cluster From Error Code.vi"("error in (no error)"=w817, "error code (0)"=w838) -> ("error out"=w819:errorcluster)  [unwired: 7 in]
                          n795 = property class="WFChart (strict)"("X Scale.Offset and Multiplier:Multiplier"=w811, "X Scale.Range:Minimum"=0.0, "X Scale.Range:Maximum"=10.0 ("y")) -> ()  [unwired: 2 in, 2 out]
                          n796 = case shown="True" w840 {
                            tunnel: w841 -> [_ w852]
                            tunnel: [w845 w849] -> w818
                            tunnel: w809 -> [_ w848]
                            tunnel: w819 -> [w845 w847]
                            tunnel: w814 -> [_ w846]
                            frame False {
                            }
                            frame True {
                              n797 = call "Write File Header.vi"("Curve Name"="VFPCURVE", "App Name"="VFP600", "error in"=w847, "Hz"=w848, "Control Mode"=w846, "File Refnum In"=w852) -> ("error out"=w849:errorcluster)  [unwired: 2 in, 1 out]
                            }
                          }
                          n798 = local read "CtrlMode"() -> (w820:u32)
                          n799 = local read "Signal"() -> (w813:refnum<k7>)
                          n800 = local read "Pstat"() -> (w821:refnum<k7>)
                          n801 = call "SigArrayInit.vi"("Signal Array"=w832, "Pstat"=w821, "Signal In"=w813, "CtrlMode"=w820, "Cycles"=w842, "Sample Rate"=w811, "error in (no error)"=w818) -> ("Pstat Out"=w836:refnum<k7>, "Signal Out"=w816:refnum<k7>, "error out"=w837:errorcluster)  [unwired: 6 in]
                          n802 = local read "GAMRYCOMLib.IGamrySignal"() -> (w833:refnum<k7>)
                          n803 = Variant To Data(error in=w837, type=w833, Variant=w816) -> (data=w834:refnum<k7>, error out=w835:errorcluster)
                          n804 = invoke class="IGamryPstat" method="SetSignal"(reference=w836, error in=w835, "Signal"=w834) -> (reference out=w808:refnum<k7>, error out=w807:errorcluster)  [unwired: 1 in, 2 out]
                          n805 = invoke class="IGamryPstat" method="InitSignal"(reference=w808, error in=w807) -> (error out=w806:errorcluster)  [unwired: 1 in, 2 out]
                          n806 = case shown="No Error" w806 {
                            tunnel: [DataAcqStates."Data Acq Setup" ("Data Acq States") DataAcqStates."STOP" ("Data Acq States")] -> w815
                            frame No Error {
                            }
                            frame Error {
                            }
                          }
                        }
                      }
                    }
                    frame "Data Acq Setup" {
                      n807 = case shown="No Error" w987 {
                        selector: w987 -> [w998 w1000]
                        tunnel: [w998 w1000] -> w988
                        frame No Error {
                          w999 = TRUE ("ForcePstatFunctionUpdate")
                          n808 = property on="ForcePstatFunctionUpdate" class="Bool (strict)"("Value (Signaling)"=w999) -> ()  [unwired: 2 in, 2 out]
                          n809 = local write "Taking Data"(w999) -> ()
                        }
                        frame Error {
                        }
                      }
                      n810 = local read "Auto Cell Switch"() -> (w989:bool)
                      n811 = local read "Pstat"() -> (w985:refnum<k7>)
                      n812 = case shown="True" w989 {
                        tunnel: w988 -> [w992 w997]
                        tunnel: [w992 w995] -> w984
                        tunnel: w985 -> [_ w993]
                        frame False {
                        }
                        frame True {
                          w996 = 1 items=["CellOff", "CellOn"] ("CellState")
                          n813 = local write "Cell State"(TRUE) -> ()
                          n814 = invoke class="IGamryPstat" method="SetCell"(reference=w993, error in=w997, "CellState"=w996) -> (error out=w995:errorcluster)  [unwired: 1 in, 3 out]
                        }
                      }
                      n815 = case shown="No Error" w984 {
                        tunnel: [DataAcqStates."Acquire Data" ("Data Acq States") DataAcqStates."STOP" ("Data Acq States")] -> w986
                        frame No Error {
                        }
                        frame Error {
                        }
                      }
                    }
                    frame "Acquire Data" {
                      # "Tell the Dtaq to Run"
                      n816 = local read "Dtaq"() -> (w1004:refnum<k7>)
                      n817 = invoke class="IGamryDtaqIv" method="Run"(reference=w1004, error in=w1003, "AutoRun"=TRUE) -> (error out=w1006:errorcluster)  [unwired: 1 in, 3 out]
                      n818 = while {
                        tunnel: [w1066] -> w1001
                        tunnel: w1006 -> [w1068]
                        stop <- w1070 stop-if-true
                        # "Overload"
                        # "If we fail here, it is likely due to a device being turned off,\nas any \"Dtaq not initialized\" errors would crop up in earlier states,\nso we'll give a more helpful error."
                        # "Im"
                        # "Vf"
                        # "Take the actual data"
                        # "Poll 2x as often as axq frequency, or X ms, whichever is larger."
                        n819 = local read "Dtaq"() -> (w1088:refnum<k7>)
                        n820 = local read "Im History"() -> (w1063:sgl[])
                        n821 = invoke class="IGamryDtaqIv" method="Cook"(reference=w1088, error in=w1068, "NumPoints"=1024) -> (error out=w1067:errorcluster, "Data"=w1086:variant)  [unwired: 2 in, 3 out]
                        n822 = local read "Acq. Frequency"() -> (w1038:dbl)
                        n823 = Array Size(array=w1063) -> (size(s)=w1059:i32)
                        n824 = case shown="True" "Pick a new filename" {
                          frame False {
                          }
                          frame True {
                            (unwired) T11."new or existing file" ("select mode (2)")
                            n825 = call <vilib>:"Open Registry Key.vi"("security access mask (KEY_READ | KEY_WRITE)"=Registry_SAM."KEY_READ", "subkey"="SOFTWARE\\Microsoft\\Windows\\CurrentVersion\\Explorer\\Shell Folders\\", "root key (HKEY_LOCAL_MACHINE)"=Registry_RtKey."HKEY_LOCAL_MACHINE") -> ("error out"=w1128:errorcluster, "refnum out"=w1126:T12)  [unwired: 7 in]
                            n826 = call-poly <vilib>:"Read Registry Value Simple.vi"("error in (no error)"=w1128, "default data"="C:\\Documents and Settings\\All Users\\Documents\\", "value"="Common Documents", "refnum"=w1126) -> ("error out"=w1127:errorcluster, "String/Binary data"=w1120:string, "refnum out"=w1125:T12)  [unwired: 2 in, 1 out]
                            n827 = call <vilib>:"Close Registry Key.vi"("error in (no error)"=w1127, "refnum"=w1125) -> ()  [unwired: 5 in, 1 out]
                            n828 = Concatenate Strings(w1120, "\\My Gamry Data\\" ("string")) -> (w1118:string)
                            n829 = String To Path(string=w1118) -> (path=w1130:path)
                            n830 = File Dialog(6:"*.txt" ("pattern"), 7:"Data File Location" ("prompt"), 9:"logfile.txt" ("default name"), 11:w1130) -> (0:w1132:errorcluster, 3:w1109:path)  [unwired: 3 in, 2 out]
                            n831 = Unbundle(w1132) -> ()  [unwired: 3 out]
                            n832 = local read "Front Panel Window:Title 2"() -> (w1113:string)
                            n833 = local write "Log File 2"(w1109) -> ()
                            n834 = call <vilib>:"Open_Create_Replace File.vi"("function (open:0)"=T8."create or replace", "file path"=w1109) -> ("refnum"=w1110:refnum<file>)  [unwired: 6 in, 3 out]
                            n835 = Path To String(path=w1109) -> (string=w1115:string)
                            n836 = local write "Log File Refnum 2"(w1110) -> ()
                            n837 = Concatenate Strings(w1113, " - " ("string"), w1115) -> (w1112:string)
                            n838 = property class="VI"("Front Panel Window:Title"=w1112) -> ()  [unwired: 2 in, 2 out]
                          }
                        }
                        n839 = Reciprocal(x=w1038) -> (1/x=w1083:dbl)
                        n840 = Subtract(x=w1059, y=16384) -> (x-y=w1061:i32)
                        n841 = Multiply(x=w1083, y=1000.0) -> (x*y=w1081:dbl)
                        n842 = Variant To Data(error in=w1067, type=sgl[][] [], Variant=w1086) -> (data=w1054:sgl[][], error out=w1052:errorcluster)
                        n843 = Array Subset(array=w1063, index=w1061) -> (w1062:sgl[])  [unwired: 1 in]
                        n844 = Index Array(array=w1054, index (row)=5) -> (element=w1053:sgl[])  [unwired: 1 in]
                        n845 = Index Array(array=w1054, index (row)=3) -> (element=w1029:sgl[])  [unwired: 1 in]
                        n846 = Index Array(array=w1054, index (row)=1) -> (element=w1011:sgl[])  [unwired: 1 in]
                        n847 = for {
                          tunnel: w1053 -> [w1145] mode=indexing
                          w1133 = cluster{u32, u32}[] [{7536640, 7536640}, {16744448, 16744448}]
                          w1134 = cluster{u32, u32}[] [{7536640, 7536640}, {16711680, 16711680}]
                          n848 = call "VFPOverloads.vi"("Overload IN"=w1145) -> ("Overloads"=w1139:T14)  [unwired: 9 in, 1 out]
                          n849 = Unbundle By Name(w1139) -> ("CA Overload"=w1143:bool)
                          n850 = Unbundle By Name(w1139) -> ("V Overload"=w1141:bool, "V ADC Railed"=w1140:bool)
                          n851 = Unbundle By Name(w1139) -> ("I Overload"=w1135:bool, "I ADC Railed"=w1138:bool)
                          n852 = local write "Control Amp Overload"(w1143) -> ()
                          n853 = Or(x=w1135, y=w1138) -> (x .or. y?=w1137:bool)
                          n854 = Or(x=w1141, y=w1140) -> (x .or. y?=w1142:bool)
                          n855 = Select(t=w1134, s=w1135, f=w1133) -> (s? t:f=w1136:cluster{u32, u32}[])
                          n856 = Select(t=w1134, s=w1141, f=w1133) -> (s? t:f=w1144:cluster{u32, u32}[])
                          n857 = property on="Current Overload" class="Bool (strict)"("Value"=w1137, "Colors [4]"=w1136) -> ()  [unwired: 2 in, 2 out]
                          n858 = property on="Voltage Overload" class="Bool (strict)"("Value"=w1142, "Colors [4]"=w1144) -> ()  [unwired: 2 in, 2 out]
                        }
                        n859 = Build Array(w1011, w1029) -> (w1030:sgl[][])
                        n860 = Divide(x=w1081, y=2.0) -> (x/y=w1079:dbl)
                        n861 = local read "Log File Refnum 2"() -> (w1031:refnum<file>)
                        n862 = local read "Start/Stop Saving"() -> (w1032:bool)
                        n863 = local read "Log File Refnum"() -> (w1075:refnum<file>)
                        n864 = local write item#33(w1030) -> ()
                        n865 = local read "Legacy Save"() -> (w1076:bool)
                        n866 = Max & Min(x=w1079, y=60.0) -> (max(x,y)=w1077:dbl)  [unwired: 1 out]
                        n867 = case shown="True" w1076 {
                          tunnel: w1075 -> [_ w1161]
                          tunnel: w1030 -> [_ w1157]
                          frame False {
                          }
                          frame True {
                            n868 = Transpose 2D Array(2D array=w1157) -> (transposed array=w1158:sgl[][])
                            n869 = Array To Spreadsheet String(array=w1158, 3:"%5g" ("format string")) -> (spreadsheet string=w1160:string)  [unwired: 1 in]
                            n870 = Write to Binary File(file (use dialog)=w1161, data=w1160, 5:FALSE ("prepend array or string size? (T)")) -> ()  [unwired: 3 in, 3 out]
                          }
                        }
                        n871 = case shown="True" w1032 {
                          tunnel: w1031 -> [_ w1108]
                          tunnel: w1030 -> [_ w1104]
                          frame False {
                          }
                          frame True {
                            n872 = Transpose 2D Array(2D array=w1104) -> (transposed array=w1105:sgl[][])
                            n873 = Array To Spreadsheet String(array=w1105, 3:"%5g" ("format string")) -> (spreadsheet string=w1107:string)  [unwired: 1 in]
                            n874 = Write to Binary File(file (use dialog)=w1108, data=w1107, 5:FALSE ("prepend array or string size? (T)")) -> ()  [unwired: 3 in, 3 out]
                          }
                        }
                        n875 = local read "Vf History"() -> (w1064:sgl[])
                        n876 = Wait (ms)(milliseconds to wait=w1077) -> ()  [unwired: 1 out]
                        n877 = Array Size(array=w1064) -> (size(s)=w1074:i32)
                        n878 = Subtract(x=w1074, y=16384) -> (x-y=w1072:i32)
                        n879 = local read "XY Graph Flipped?"() -> (w1057:bool)
                        n880 = Array Subset(array=w1064, index=w1072) -> (w1069:sgl[])  [unwired: 1 in]
                        n881 = property on="Recording IV" class="Bool (strict)"() -> ("Value"=w1026:bool)  [unwired: 2 in, 2 out]
                        n882 = Build Array (concatenate)(w1069, w1011) -> (w1046:sgl[])
                        n883 = Build Array (concatenate)(w1062, w1029) -> (w1043:sgl[])
                        n884 = case shown="True" w1026 {
                          tunnel: w1011 -> [w1092 w1099]
                          tunnel: w1029 -> [w1093 w1096]
                          tunnel: [w1092 w1095] -> w1028
                          tunnel: [w1093 w1094] -> w1027
                          frame False {
                          }
                          frame True {
                            n885 = feedback #1() -> (w1097:sgl[])  [unwired: 1 in]
                            n886 = Build Array (concatenate)(w1097, w1096) -> (w1094:sgl[])
                            n887 = feedback-in #1(w1094) -> ()
                            n888 = feedback #2() -> (w1098:sgl[])  [unwired: 1 in]
                            n889 = Build Array (concatenate)(w1098, w1099) -> (w1095:sgl[])
                            n890 = feedback-in #2(w1095) -> ()
                          }
                        }
                        n891 = local write "Vf History"(w1046) -> ()
                        n892 = case shown="False" w1057 {
                          tunnel: w1046 -> [w1148 w1151]
                          tunnel: w1043 -> [w1147 w1150]
                          tunnel: [w1146 w1149] -> w1058
                          frame True {
                            n893 = Build Cluster Array(w1147, w1148) -> (w1146:cluster{sgl, sgl}[])
                          }
                          frame False {
                            n894 = Build Cluster Array(w1151, w1150) -> (w1149:cluster{sgl, sgl}[])
                          }
                        }
                        n895 = local write "Im History"(w1043) -> ()
                        n896 = Array Size(array=w1046) -> (size(s)=w1049:i32)
                        n897 = Array Size(array=w1043) -> (size(s)=w1045:i32)
                        n898 = Subtract(x=w1049, y="Smoothing Parameter") -> (x-y=w1048:i32)
                        n899 = Subtract(x=w1045, y="Smoothing Parameter") -> (x-y=w1044:i32)
                        n900 = local read "Start/Stop"() -> (w1091:bool)
                        n901 = Array Subset(array=w1046, index=w1048, length="Smoothing Parameter") -> (w1047:sgl[])
                        n902 = Array Subset(array=w1043, index=w1044, length="Smoothing Parameter") -> (w1042:sgl[])
                        n903 = local read "DataDone?"() -> (w1089:bool)
                        n904 = local write "I vs. V"(w1058) -> ()
                        n905 = call-poly <vilib>:"Mean.vi"("X"=w1047) -> ("mean"=w1051:dbl)  [unwired: 1 out]
                        n906 = Not(x=w1091) -> (.not. x?=w1090:bool)
                        n907 = call-poly <vilib>:"Mean.vi"("X"=w1042) -> ("mean"=w1050:dbl, "error"=w1035:i32)
                        n908 = Or(x=w1089, y=w1090) -> (x .or. y?=w1071:bool)
                        n909 = Multiply(x=w1035, y=1000000000) -> (x*y=w1034:i32)
                        n910 = Divide(x=w1051, y=w1050) -> (x/y=w1040:dbl)
                        n911 = call <vilib>:"Find First Error.vi"("error in (no error)"=w1052) -> ("error out"=w1065:errorcluster, "error?"=w1041:bool)  [unwired: 3 in]
                        n912 = case shown="True" w1026 {
                          tunnel: w1028 -> [_ w1101]
                          tunnel: w1027 -> [_ w1102]
                          frame False {
                          }
                          frame True {
                            n913 = Bundle("type"=w1102, "type"=w1101) -> (→"XY Graph":cluster{"type":sgl[], "type":sgl[]})  [unwired: 1 in]
                          }
                        }
                        n914 = case shown="No Error" w1065 {
                          selector: w1065 -> [w1152 w1154]
                          tunnel: [w1152 w1153] -> w1066
                          frame No Error {
                          }
                          frame Error {
                            n915 = Bundle By Name(cluster=w1154, "source"="Data Acq\n\nPlease confirm that your device has \nnot been disabled or disconnected.") -> (w1153:errorcluster)
                          }
                        }
                        n916 = local write "Current(nA)"(w1034) -> ()
                        n917 = Or(x=w1041, y=w1071) -> (x .or. y?=w1070:bool)
                        n918 = Divide(x=w1040, y=1000000) -> (x/y=w1025:dbl)
                        n919 = local write "Resistance (MOhm)"(w1025) -> ()
                        n920 = call "calculate_resistance.vi"("Bare Resistance (MOhm)"="Bare Resistance \n(MOhm)", "Live Resistance"=w1025, "Solution Conductance \nS/m"="Solution Conductance", "Sealed Resistance (MOhm)"="Sealed Resistance\n(MOhm)", "Membrane Thickness (nm)"="Membrane Thickness \n(nm)", "Override"="Enable Section", "Desired Pore Size (nm)"="Desired Pore Size (nm)", "Applied Voltage (V)"="Applied Voltage (V)") -> ("Boolean"=w1018:bool, "Target Resistance (MOhm)"=→"Target Resistance \n(MOhm)":dbl, "Capillary Resistance"=→"Capillary Resistance":dbl, "Capillary Diameter (nm)"=→"Capillary Diameter":dbl, "Membrane-Solution Resistivity"=→"Membrane-Solution Resistivity":dbl, "Pore Resistance"=→"Pore Resistance":dbl, "Membrane Resistance (MOhm)"=→"Membrane Resistance (MOhm)":dbl, "Target Golovochenko  (MOhm)"=→"Target Golovochenko  (MOhm)":dbl)  [unwired: 4 in]
                        n921 = local write "Start/Stop"(w1018) -> ()
                      }
                      n922 = case shown="No Error" w1001 {
                        tunnel: [DataAcqStates."Cleanup" ("Data Acq States") DataAcqStates."STOP" ("Data Acq States")] -> w1002
                        frame No Error {
                        }
                        frame Error {
                        }
                      }
                    }
                    frame "Cleanup" {
                      n923 = local read "Device Gone"() -> (w1169:bool)
                      n924 = local read "Auto Cell Switch"() -> (w1171:bool)
                      n925 = Not(x=w1169) -> (.not. x?=w1172:bool)
                      n926 = And(x=w1171, y=w1172) -> (x .and. y?=w1173:bool)
                      n927 = local read "Pstat"() -> (w1167:refnum<k7>)
                      n928 = case shown="True" w1173 {
                        tunnel: [w1187 w1192] -> w1174
                        tunnel: w1168 -> [w1187 w1190]
                        tunnel: w1167 -> [_ w1189]
                        frame False {
                        }
                        frame True {
                          w1188 = 0 items=["CellOff", "CellOn"] ("CellState")
                          n929 = local write "Cell State"(FALSE) -> ()
                          n930 = invoke class="IGamryPstat" method="SetCell"(reference=w1189, error in=w1190, "CellState"=w1188) -> (error out=w1192:errorcluster)  [unwired: 1 in, 3 out]
                        }
                      }
                      n931 = local read "Dtaq"() -> (w1170:refnum<k7>)
                      n932 = invoke class="IGamryDtaqIv" method="Stop"(reference=w1170, error in=w1174) -> (reference out=w1164:refnum<k7>, error out=w1163:errorcluster)  [unwired: 1 in, 1 out]
                      n933 = while {
                        shift-right: [w1176] -> _
                        shift-left: w1164 -> [w1181]
                        shift-right: [w1177] -> w1162
                        shift-left: w1163 -> [w1180]
                        stop <- w1178 stop-if-true
                        n934 = invoke class="IGamryDtaqIv" method="Cook"(reference=w1181, error in=w1180, "NumPoints"=1024) -> (reference out=w1176:refnum<k7>, error out=w1177:errorcluster, "NumPoints"=w1179:i32)  [unwired: 2 in, 2 out]
                        n935 = Equal To 0?(x=w1179) -> (x = 0?=w1178:bool)
                      }
                      n936 = case shown="No Error" w1162 {
                        selector: w1162 -> [w1183 w1184]
                        tunnel: [w1183 w1184] -> w1165
                        frame No Error {
                          n937 = local write "Taking Data"(FALSE) -> ()
                        }
                        frame Error {
                        }
                      }
                      n938 = case shown="No Error" w1165 {
                        tunnel: [DataAcqStates."STOP" ("Data Acq States") DataAcqStates."STOP" ("Data Acq States")] -> w1166
                        frame No Error {
                        }
                        frame Error {
                        }
                      }
                    }
                    frame "STOP" {
                      w1198 = u8 0 ("Disabled")
                      w1193 = FALSE
                      w1201 = FALSE ("Begin")
                      # "Enable menu items"
                      # "Reset Buttons"
                      n939 = local write "Start/Stop"(w1201) -> ()
                      n940 = local write "DataDone?"(w1201) -> ()
                      n941 = local write "Device Gone"(w1201) -> ()
                      n942 = property on="Device" class="Ring (strict)"("Disabled"=w1198) -> ()  [unwired: 2 in, 2 out]
                      n943 = property on="CtrlMode" class="Ring (strict)"("Disabled"=w1198) -> ()  [unwired: 2 in, 2 out]
                      n944 = property on="Ich Range" class="Ring (strict)"("Disabled"=w1198) -> ()  [unwired: 2 in, 2 out]
                      n945 = local write "Current Overload"(w1193) -> ()
                      n946 = local write "Control Amp Overload"(w1193) -> ()
                      n947 = local write "Voltage Overload"(w1193) -> ()
                      n948 = local read "Legacy Save"() -> (w1208:bool)
                      n949 = local read "CtrlMode"() -> (w1197:u32)
                      n950 = property on="Vch Range" class="Ring (strict)"("Disabled"=w1198) -> ()  [unwired: 2 in, 2 out]
                      n951 = property on="Acq. Frequency" class="DigNum (strict)"("Disabled"=w1198) -> ()  [unwired: 2 in, 2 out]
                      n952 = property on="Legacy Save" class="Bool (strict)"("Disabled"=w1198) -> ()  [unwired: 2 in, 2 out]
                      n953 = case shown="1, Default" w1197 {
                        frame 1, Default {
                          w1209 = u8 0 ("Disabled")
                          n954 = property on="I/E Range" class="Ring (strict)"("Disabled"=w1209) -> ()  [unwired: 2 in, 2 out]
                          n955 = property on="I/E Autorange" class="Bool (strict)"("Disabled"=w1209) -> ()  [unwired: 2 in, 2 out]
                        }
                        frame 0 {
                          w1210 = u8 2 ("Disabled")
                          n956 = property on="I/E Range" class="Ring (strict)"("Disabled"=w1210) -> ()  [unwired: 2 in, 2 out]
                          n957 = property on="I/E Autorange" class="Bool (strict)"("Disabled"=w1210) -> ()  [unwired: 2 in, 2 out]
                        }
                      }
                      n958 = case shown="True" w1208 {
                        tunnel: [w1217 w1219] -> w1205
                        tunnel: w1204 -> [w1217 w1218]
                        frame False {
                        }
                        frame True {
                          n959 = local read "Log File Refnum"() -> (w1220:refnum<file>)
                          n960 = Close File(refnum=w1220, error in=w1218) -> (error out=w1219:errorcluster)  [unwired: 1 out]
                        }
                      }
                      n961 = local read "DataDone Callback"() -> (w1206:refnum<k27>)
                      n962 = property class="App"() -> ("Application:Kind"=w1199:T3)  [unwired: 2 in, 2 out]
                      n963 = case shown="\"Run Time System\", Default" w1199 {
                        tunnel: [w1211 w1212] -> w1200
                        frame "Development System" {
                          w1211 = T2 1 items=["no dialog", "OK message", "continue or stop message", "OK message + warnings", "continue/stop + warnings"] ("type of dialog (OK msg:1)")
                        }
                        frame "Run Time System", Default {
                          w1212 = T2 1 items=["no dialog", "OK message", "continue or stop message", "OK message + warnings", "continue/stop + warnings"] ("type of dialog (OK msg:1)")
                        }
                      }
                      n964 = Not A Number/Path/Refnum?(number/path/refnum=w1206) -> (NaN/Path/Refnum?=w1207:bool)
                      n965 = case shown="False" w1207 {
                        tunnel: w1206 -> [w1215 _]
                        tunnel: w1205 -> [w1214 w1216]
                        tunnel: [w1213 w1216] -> w1196
                        frame False {
                          n966 = Unregister For Events(event registration refnum=w1215, error in=w1214) -> (error out=w1213:errorcluster)
                        }
                        frame True {
                        }
                      }
                      n967 = local read "[user-defined descriptions]"() -> (w1202:string[])
                      n968 = local read "[user-defined codes]"() -> (w1194:u32[])
                      n969 = call <vilib>:"General Error Handler.vi"("[user-defined codes]"=w1194, "[user-defined descriptions]"=w1202, "type of dialog (OK msg:1)"=w1200, "error in (no error)"=w1196) -> ("error out"=w1195:errorcluster)  [unwired: 7 in, 4 out]
                    }
                  }
                  n970 = Wait (ms)(milliseconds to wait=u32 150) -> ()  [unwired: 1 out]
                  n971 = Equal?(x=w712, y=DataAcqStates."STOP" ("Data Acq States")) -> (x = y?=w713:bool)
                }
              }
            }
          }
          event Timeout {
            n972 = event-data() -> ()  [unwired: 1 in, 3 out]
          }
        }
      }
    }
    frame #3 {
      w1224 = 0.0
      w1221 = u8 0 ("Disabled")
      w1222 = u16 0 items=[""] ("I/E Range")
      w1229 = 0 ("First I/E Range")
      w1223 = string[] [] ("Strings []")
      w1227 = FALSE ("Begin")
      # "Reset Buttons and Variables"
      n973 = local write "Section"("" ("Section")) -> ()
      n974 = local write "Close"(w1227) -> ()
      n975 = property on="Vch Range" class="Ring (strict)"("Strings []"=w1223, "Value"=w1222, "Disabled"=w1221) -> ()  [unwired: 2 in, 2 out]
      n976 = property on="Device" class="Ring (strict)"("Strings []"=w1223, "Value"=w1222, "Disabled"=w1221) -> ()  [unwired: 2 in, 2 out]
      n977 = property on="Ich Range" class="Ring (strict)"("Strings []"=w1223, "Value"=w1222, "Disabled"=w1221) -> ()  [unwired: 2 in, 2 out]
      n978 = property on="Vch Filter" class="Ring (strict)"("Strings []"=w1223, "Value"=w1222, "Disabled"=w1221) -> ()  [unwired: 2 in, 2 out]
      n979 = property on="Ich Filter" class="Ring (strict)"("Strings []"=w1223, "Value"=w1222, "Disabled"=w1221) -> ()  [unwired: 2 in, 2 out]
      n980 = property on="I/E Range" class="Ring (strict)"("Strings []"=w1223, "Value"=w1222, "Disabled"=w1221) -> ()  [unwired: 2 in, 2 out]
      n981 = property on="CA Speed" class="Ring (strict)"("Strings []"=w1223, "Value"=w1222, "Disabled"=w1221) -> ()  [unwired: 2 in, 2 out]
      n982 = property on="CtrlMode" class="Ring (strict)"("Value"=w1222, "Disabled"=w1221) -> ()  [unwired: 2 in, 2 out]
      n983 = property on="I/E Autorange" class="Bool (strict)"("Disabled"=w1221) -> ()  [unwired: 2 in, 2 out]
      n984 = property on="Vch Offset" class="DigNum (strict)"("Value"=w1224, "Disabled"=w1221) -> ()  [unwired: 2 in, 2 out]
      n985 = property on="Ich Offset" class="DigNum (strict)"("Value"=w1224, "Disabled"=w1221) -> ()  [unwired: 2 in, 2 out]
      n986 = local write "Device"(w1229) -> ()
      n987 = local write "Start/Stop"(w1227) -> ()
      n988 = local write "I/E Autorange"(w1227) -> ()
      n989 = local write "Vch Autorange"(w1227) -> ()
      n990 = local write "Ich Autorange"(w1227) -> ()
      n991 = local write "Cell State"(w1227) -> ()
      n992 = local write "VchOffsetEnable"(w1227) -> ()
      n993 = local write "IchOffsetEnable"(w1227) -> ()
      n994 = local write "Device List Change"(w1227) -> ()
      n995 = local write "First I/E Range"(w1229) -> ()
      n996 = local read "Device List Change Callback"() -> (w1226:refnum<k27>)
      n997 = property on="I/E Range" class="Ring (strict)"("Strings []"=w1223, "Value"=w1222, "Disabled"=w1221) -> ()  [unwired: 2 in, 2 out]
      n998 = Not A Number/Path/Refnum?(number/path/refnum=w1226) -> (NaN/Path/Refnum?=w1225:bool)
      n999 = case shown="False" w1225 {
        tunnel: w1226 -> [w1230 _]
        frame False {
          n1000 = Unregister For Events(event registration refnum=w1230) -> ()  [unwired: 1 in, 1 out]
        }
        frame True {
        }
      }
    }
  }
  "Confirm Exit?" <- FALSE
  "Version" <- "5.62" ("Version")
  "Voltage Overload" <- w1
  "Current Overload" <- w1
  "Control Amp Overload" <- w1
